vi "Main VERSION 2.0.vi"() -> ()   [LabVIEW 2017]
doc: "This Continuous Measurement sample project is based on the Queued Message Handler template.\n\nThe Event Handling Loop generates messages based on user interface actions.\n\nThe Message Handling Loop processes messages generated by the Event Handling Loop, or by other messages. There are also Acquisition and Logging message handling loop subVIs, and a chart updating loop."
uses:
  support/libs/Signal Selector/Selection Folder/Selection.xctl
  <vilib>/Math Plots/3D Math Plots/3D Surface/3D Surface XCtrl/3D Surface.xctl
  <vilib>/Math Plots/3D Math Plots/3D Surface/3D Surface Datatype/3D Surface Datatype.lvclass
  controls/UI Data.ctl
  support/libs/PMU Buffer/Buffer DATA cluster.ctl
  controls/UI State.ctl
  acquisition/Acquisition Settings.ctl
  acquisition/Acquisition State.ctl
  support/libs/CSV Reader/Mode CSV reader.ctl
  logging/Logging Configuration.ctl
  logging/Logging State.ctl
  support/libs/PMU Buffer/Buffer Settings.ctl
  processing/Processing Settings.ctl
  processing/Display Data B.ctl
  processing/Display Data A.ctl
  <vilib>/Math Plots/3D Math Plots/3D Plot/3D Plot Datatype/3D Plot Datatype.lvclass
  <vilib>/Utility/error.llb/DialogType.ctl
  support/libs/PMU Buffer/Buffer state.ctl
  support/settings/Settings.ctl
  b850246f-c621-4cc8-8cdb-6c63488b8d16.vi
  d6c7b380-5ef8-42a0-a533-ce26cb609579.vi
  5953c9e4-e6ed-48ce-a3e3-f4074e595e54.vi
  308fbb3a-e3c1-4651-8528-14e79cd65b6c.vi
  fb94752c-021c-42e0-8cca-361a15baff7d.vi
  17f702fa-b3ef-4227-89b6-1808d4fdff79.vi
  support/Message Queue/Enqueue Message (Single).vi
  <vilib>/S3DK/PMU Recorder Light/PRL Channel Selector.vi
  support/settings/Get Config File Path.vi
  <vilib>/Utility/xml.llb/Read From XML File.vi
  <vilib>/Utility/xml.llb/Read From XML File(string).vi
  <vilib>/Utility/xml.llb/Write to XML File.vi
  <vilib>/Utility/xml.llb/Write to XML File(string).vi
  <vilib>/Utility/error.llb/Error Cluster From Error Code.vi
  <vilib>/ErrorRing/Error Ring.xnode
  acquisition/Acquisition.lvlib
  logging/Logging.lvlib
  support/User Event - Stop/User Event - Stop.lvlib
  support/Message Queue/Message Queue.lvlib
  support/settings/Settings Dialog.vi
  support/settings/Settings.lvlib
  processing/Processing.lvlib
  support/libs/PMU Buffer/PMU data buffer.lvlib
  <vilib>/S3DK/PMU Recorder Light/PMU Recorder Light.lvlib
  support/libs/Signal Selector/Signal Selector.lvlib
panel:
  in  "Data Selector":bool
  in  "PRL Visible":bool
  out "Display 2":bool
  out "Buffer Active":bool
  out "Config File":bool
  out "Connected":bool
  out "Error":bool
  out "Processing":bool=TRUE
  out "Display":bool
  out "Acquisition":bool=TRUE
  out "Events":bool=TRUE
  out "Buffer":bool
  out "UI Control":bool
  in  "Tab Control":T1(tab)
  out "ARMA Transfer Function":picture
  out "Critical Damping [%]":dbl
  out "Critical Frequency [Hz]":dbl
  out "Estimated Complex Plane":cluster{dbl[], dbl[]}(graph)
  out "Damping ratio evolution":dbl[][](graph)
  out "Real-time data":waveform(dbl)(graph)={"t0"=timestamp(3467964116.0127993 s since 1904-01-01), "dt"=0.02, "Y"=array[30000 elements]}
  out "Preprocessed data":waveform(dbl)(graph)={"t0"=timestamp(3467964116.0127993 s since 1904-01-01), "dt"=0.2, "Y"=array[3000 elements]}
  out "Spectrogram":refnum<class "3D Plot Datatype.lvclass">[](xcontrol)
  out "Spectrum":cluster{"f0":dbl, "df":dbl, "S(f)":dbl[]}(graph)={"f0"=0.0, "df"=0.0048828125, "S(f)"=[]}
  out "Picture 9":picture
  out "Picture 8":picture
  out "Picture 7":picture
  out "Picture 6":picture
  out "Picture 5":picture
  out "Picture 4":picture
  out "Picture 3":picture
  out "Picture 2":picture
  out "Picture 1":picture
  out "Std of Damping":dbl[](array[numeric])
  out "Mean Damping [%]":dbl[](array[numeric])
  out "Frequency[Hz]":dbl[](array[numeric]) format="%.4f"
  out "Damping Ratio [%]":dbl[](array[numeric]) format="%.4f"
  out "Complex Poles":cdb[](array[numeric]) format="%.4f"
  in  "Selection":cluster{"Type":T2, "Index(es)":i32[]}[](xcontrol)
  in  "Settings":bool
  in  "Start":bool
  in  "Stop":bool
  out "Status":string
  in  "Exit":bool
  # "Continuous Measurement Data Logger"
  # "MA\n_______\n\n   AR"
  # "If you hit the bottom button, you will see the same chart as the one \non the Spectrum graph"
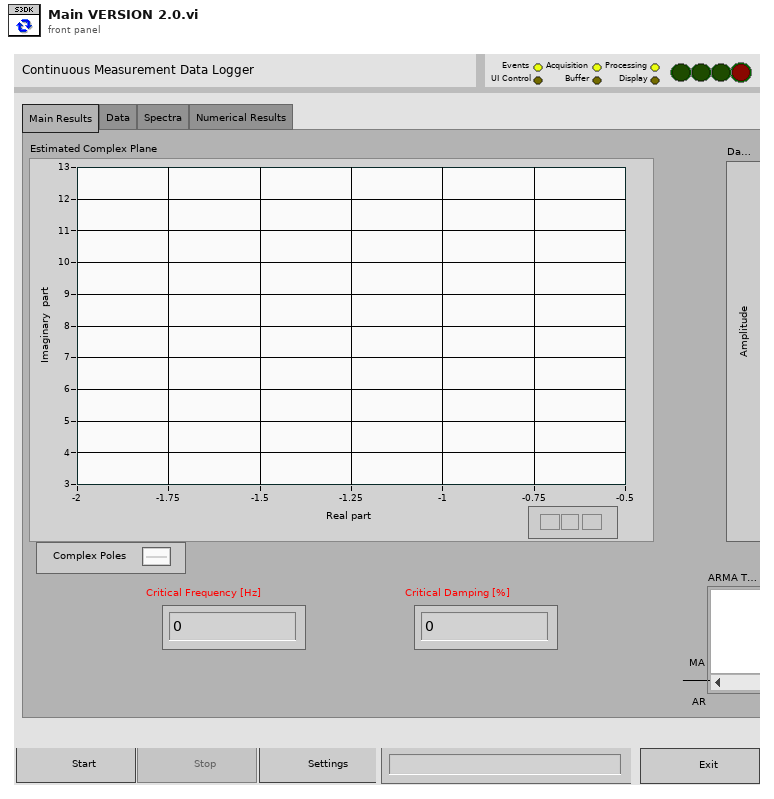
[diagram p1: front panel]
types:
  T1 = enum32{"Main Results", "Data", "Spectra", "Numerical Results"}
  T2 = typedef "Selection.xctl/Signal types.ctl" = enum16{"Disable", "Frequency", "Phasor Mag", "Phasor Ang", "Angle Diff", "P", "Q"}
  T3 = typedef "Display Data A.ctl" = cluster{"Real-time data":waveform(dbl), "Preprocessed data":waveform(dbl), "ARMA Transfer Function":picture, "Spectrogram":refnum<class "3D Plot Datatype.lvclass">[], "Spectrum":cluster{"f0":dbl, "df":dbl, "S(f)":dbl[]}, "Parcel Length (SDK or Simulation)":i32}
  T4 = typedef "Display Data B.ctl" = cluster{"Damping ratio evolution":dbl[][], "Estimated Complex Plane":cluster{dbl[], dbl[]}, "Critical Frequency [Hz]":dbl, "Critical Damping [%]":dbl, " Complex Poles":cdb[], "Damping Ratio [%]":dbl[], " Frequency[Hz]":dbl[], "Mean Damping [%]":dbl[], "Pictures":picture[], "Std of Damping":dbl[]}
  T5 = typedef "Processing.lvlib/Processing Settings.ctl" = cluster{"Settings":string, "Parameters":T6, "Refresh Rate":u32}
  T6 = typedef "PMU data buffer.lvlib/Buffer Settings.ctl" = cluster{"Index":i32, "Size":i32, "Samples":i32, "Ordered ?":bool}
  T7 = typedef "Logging.lvlib/Logging Configuration.ctl" = cluster{"Logging State":T8, "Settings":string, "Buffer":T6}
  T8 = typedef "Logging.lvlib/Logging State.ctl" = enum16{"Idle", "Logging"}
  T9 = typedef "Acquisition.lvlib/Acquisition Settings.ctl" = cluster{"State":T10, "Settings":string, "Online":bool, "S3DK":cluster{"Signals":cluster{"Phasor":string[], "Analog":string[], "Digital":string[]}}, "CSV":cluster{"Index":i32, "Parcel Length":i32, "EOF?":bool, "Config":cluster{"Mode":T11, "delimiter (\\t)":string, "Path":path, "Rectangular?":bool}}}
  T10 = typedef "Acquisition.lvlib/Acquisition State.ctl" = enum16{"Idle", "Idle S3DK", "Acquiring S3DK", "Idle CSV", "Acquiring CSV"}
  T11 = typedef "Mode CSV reader.ctl" = enum16{"Full timestamp", "Relative Time", "Seconds Time", "Nanoseconds Time"}
  T12 = typedef "UI State.ctl" = enum16{"Idle", "Acquiring and Logging", "Waiting for Exit", "Waiting for Exit (Acq Stopped)", "Waiting for Exit (Log Stopped)", "Waiting for Stop", "Waiting for Stop (Acq Stopped)", "Waiting for Stop (Log Stopped)"}
  T13 = typedef "PMU data buffer.lvlib/Buffer DATA cluster.ctl" = cluster{timestamp, csg[], sgl[]}
  T14 = typedef "UI Data.ctl" = cluster{"Start Ref":refnum<vi>, "Stop Ref":refnum<vi>, "Settings Ref":refnum<vi>, "Exit Ref":refnum<vi>, "Status Ref":refnum<vi>, "Data Ref":refnum<vi>, "Data Selector":refnum<vi>, "PRL Visible":refnum<vi>}
  T15 = typedef "Message Queue.lvlib/All Message Queues.ctl" = cluster{"UI":refnum<queue>, "Acquisition":refnum<queue>, "Logging":refnum<queue>, "Processing":refnum<queue>}
  T16 = typedef "PMU data buffer.lvlib/Buffer state.ctl" = enum16{"Init", "Change Size", "Flush", "Exit", "Add", "Get", "Hist_Toggle", "Add_Serv"}
  T17 = typedef "DialogType.ctl" = u16
  T18 = typedef "Mode Est Processing Settings.ctl" = cluster{"Low-Pass Filter Order":i32, "Downsampling Ratio":dbl, "LPF Cut-off Frequency [Hz]":dbl, "Sampling Frequency (Hz)":dbl, "Parcel Length":i32, "Detrend Cut-off Frequency (Hz)":dbl, "AR Order":i32, "MA Order ":i32, "Lower Frequency [Hz]":dbl, "Upper Frequency [Hz]":dbl, "Upper Damping [%]":dbl, "Lower Damping [%]":dbl, "Std Threshold":dbl, "Length of Spectra [s]":dbl, "Refresh Rate [s]":i32, "Number of critical modes":i32}
  T19 = typedef "PMU data buffer.lvlib/Buffer DATA OUT ordered.ctl" = cluster{"Timestamp":timestamp[], "Phasor":csg[][], "Analog":sgl[][]}
  T20 = enum16{"Run", "Startup", "Get Status", "Pause", "Continue", "Shutdown", "Abort", "Open Panel", "Close Panel"}
  T21 = enum32{"Invalid", "Standard", "Closed", "Hidden", "Minimized", "Maximized"}
  T22 = typedef "Settings.lvlib/Settings.ctl" = cluster{"Acquisition":T9, "Logging":T7, "Processing":T5}
  T23 = cluster{"[0]":variant, "[1]":variant, "[2]":variant}
  T24 = typedef "Terminal Data.ctl" = cluster{"Spreadsheet":path, "Terminal ID":u32, "Terminal Name":string}
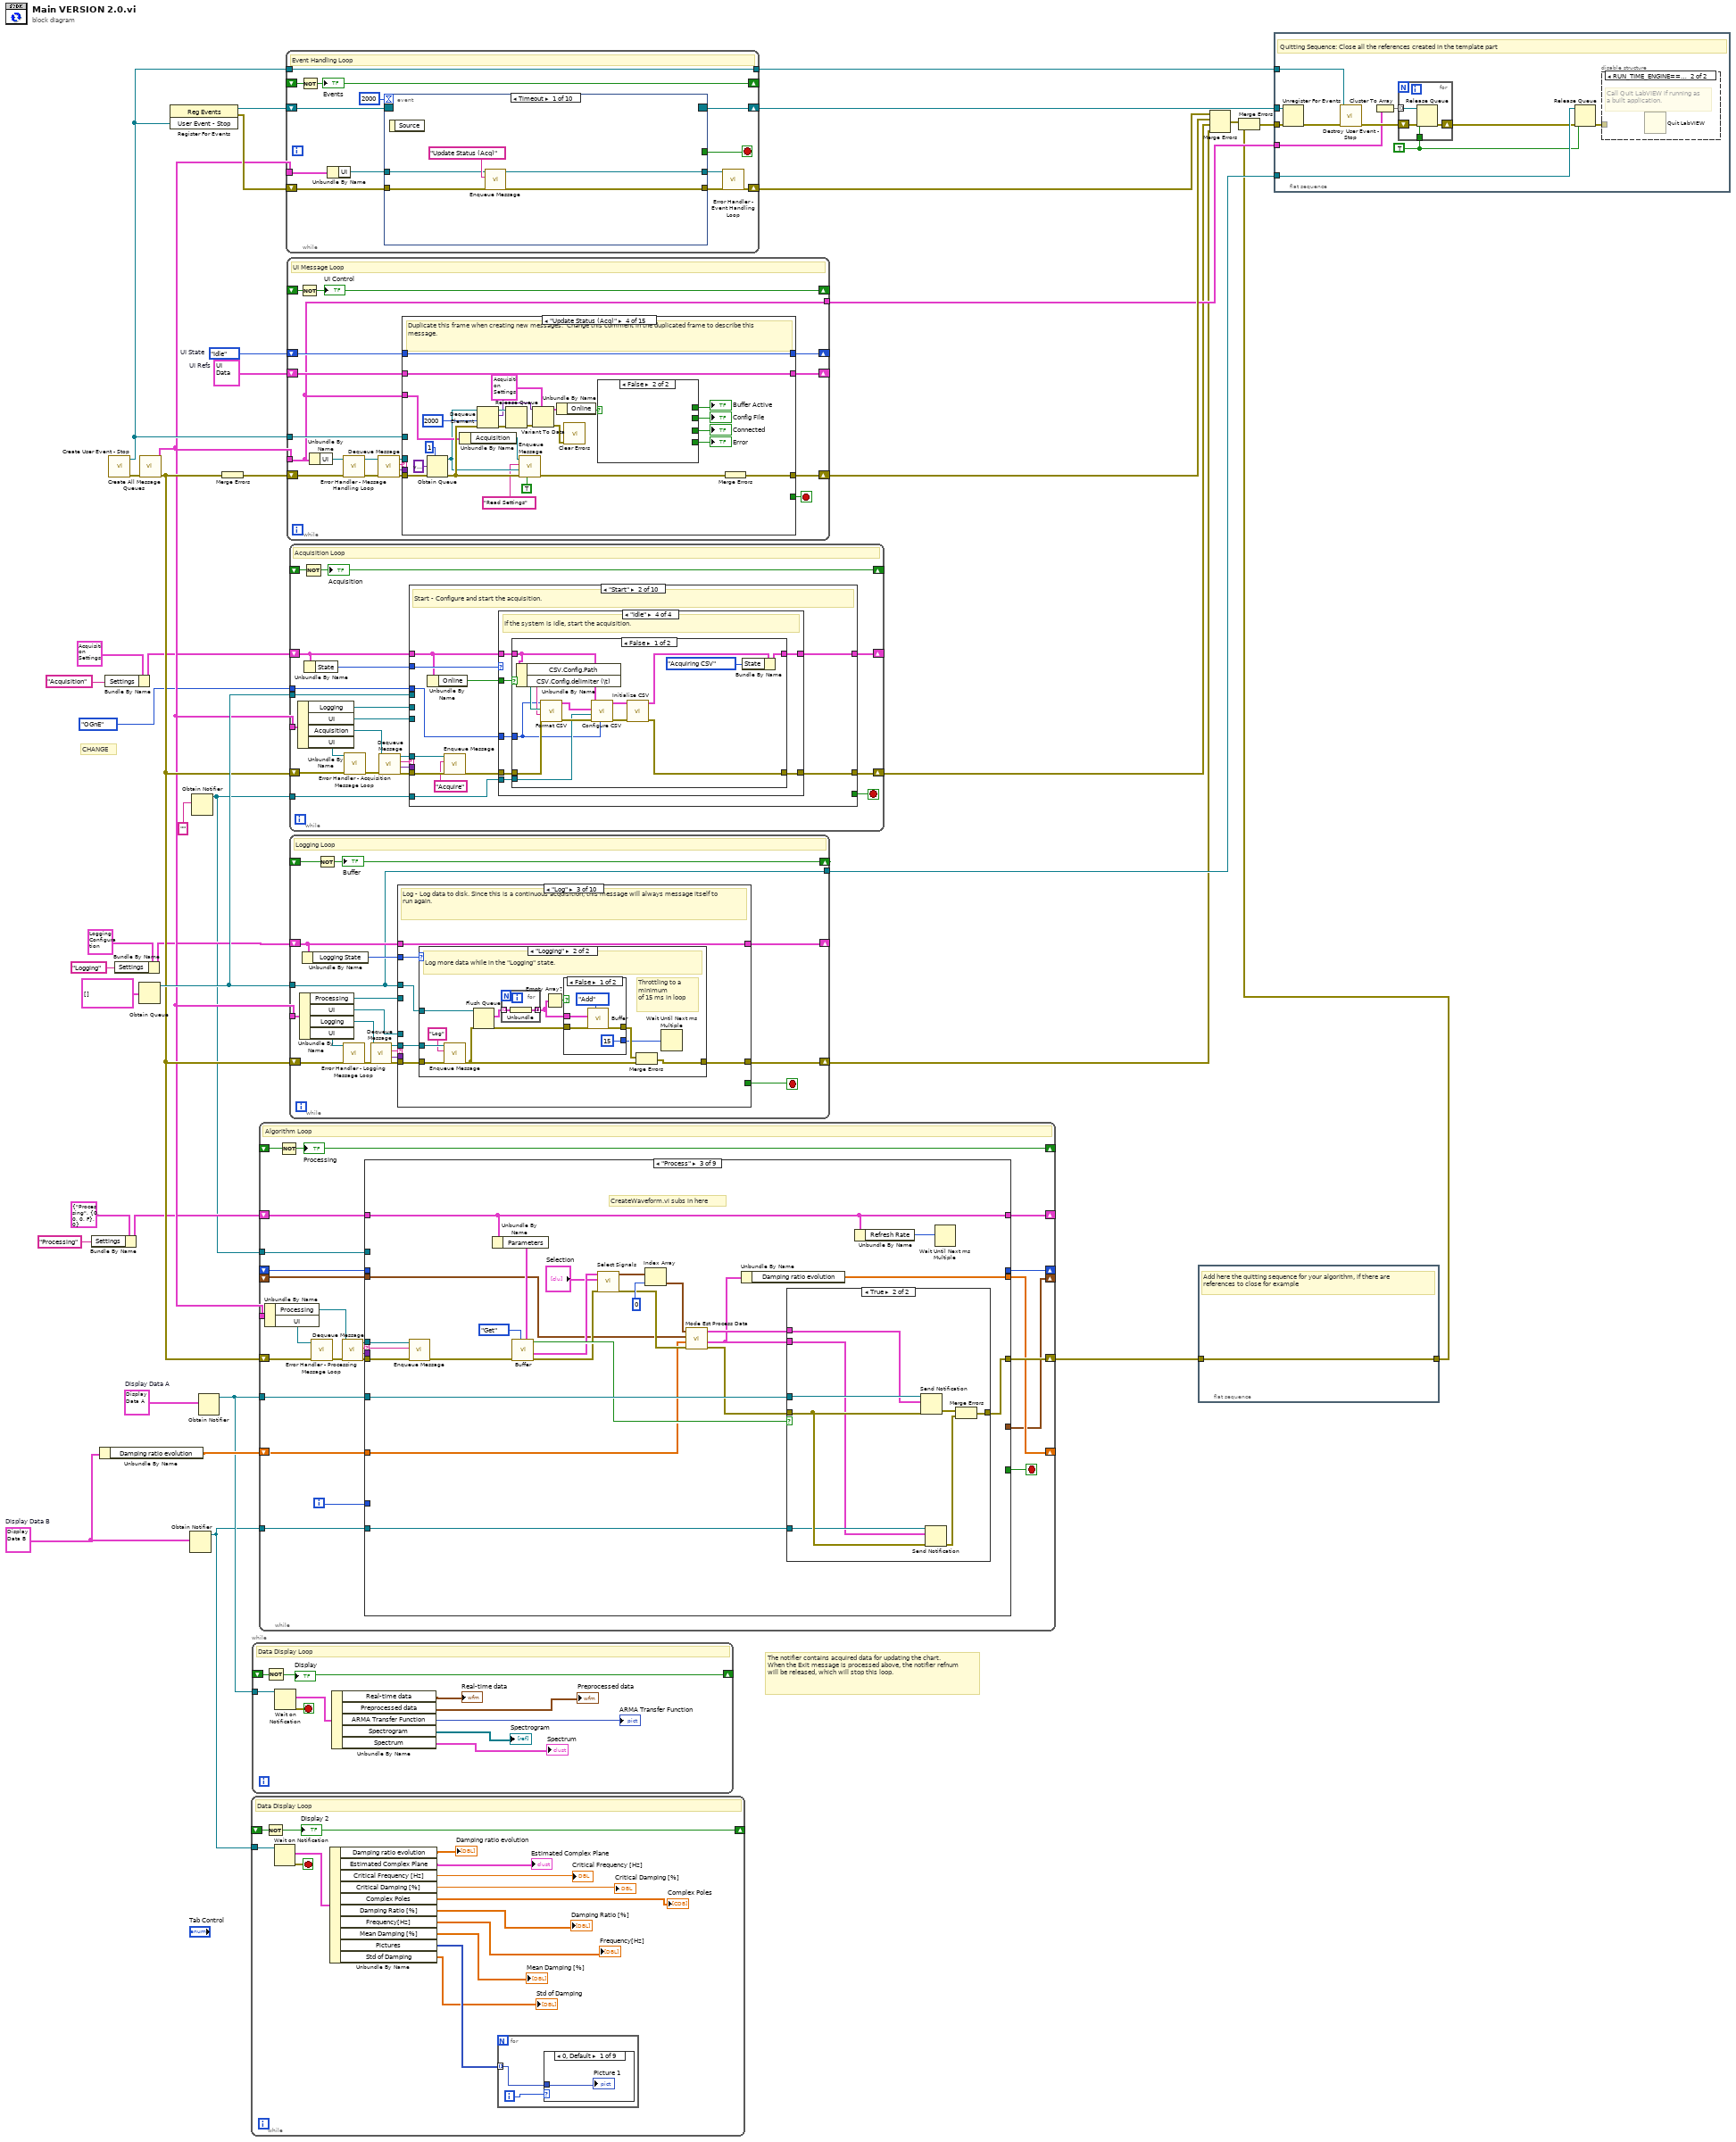
[diagram p0: block diagram]
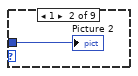
[diagram p2: hidden frame]
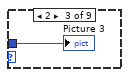
[diagram p3: hidden frame]
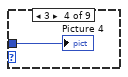
[diagram p4: hidden frame]
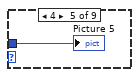
[diagram p5: hidden frame]
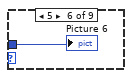
[diagram p6: hidden frame]
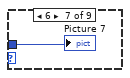
[diagram p7: hidden frame]
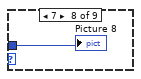
[diagram p8: hidden frame]
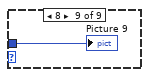
[diagram p9: hidden frame]
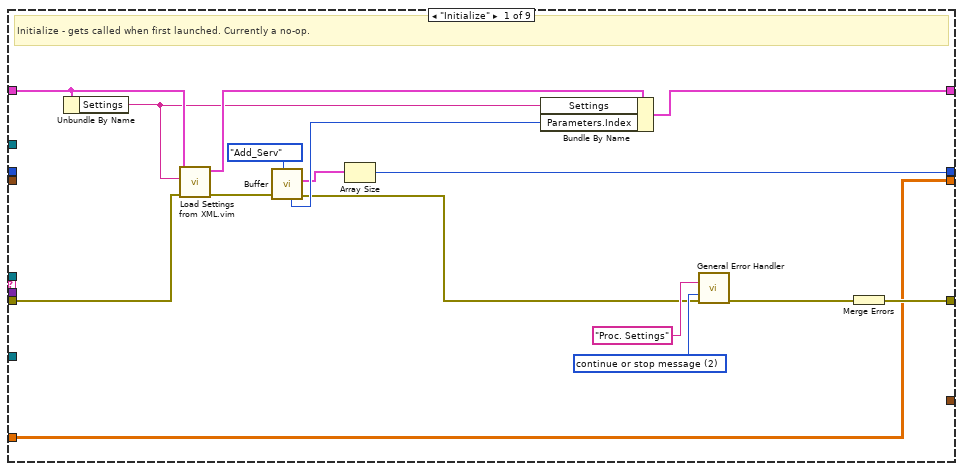
[diagram p11: hidden frame]
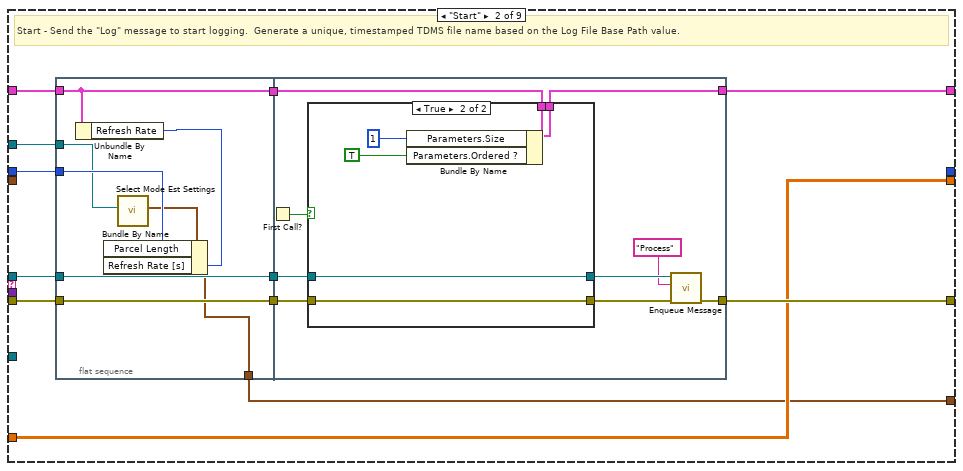
[diagram p12: hidden frame]
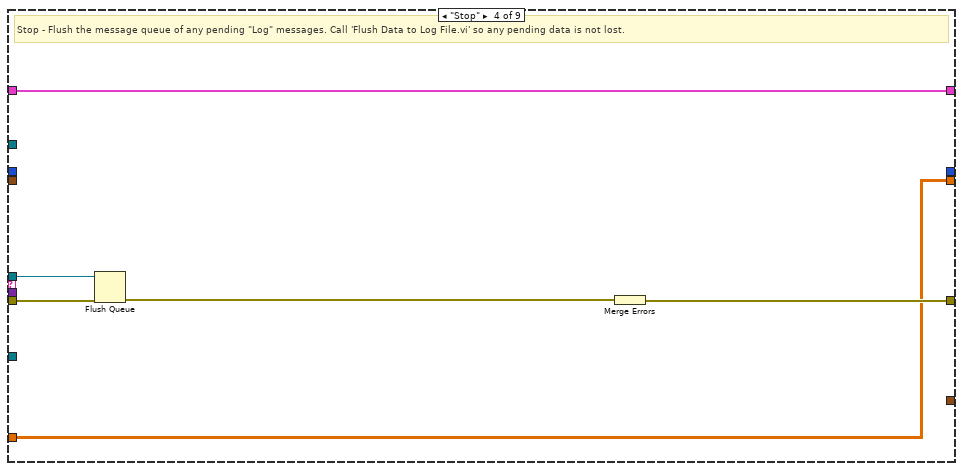
[diagram p15: hidden frame]
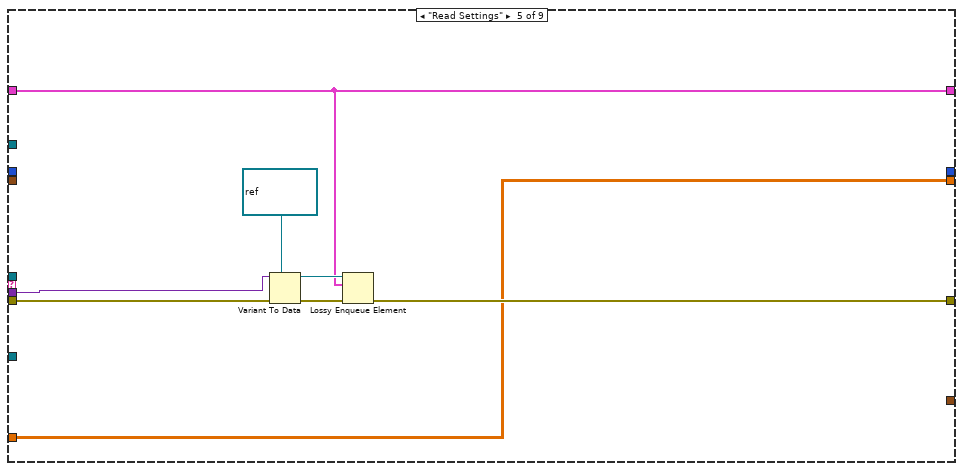
[diagram p16: hidden frame]
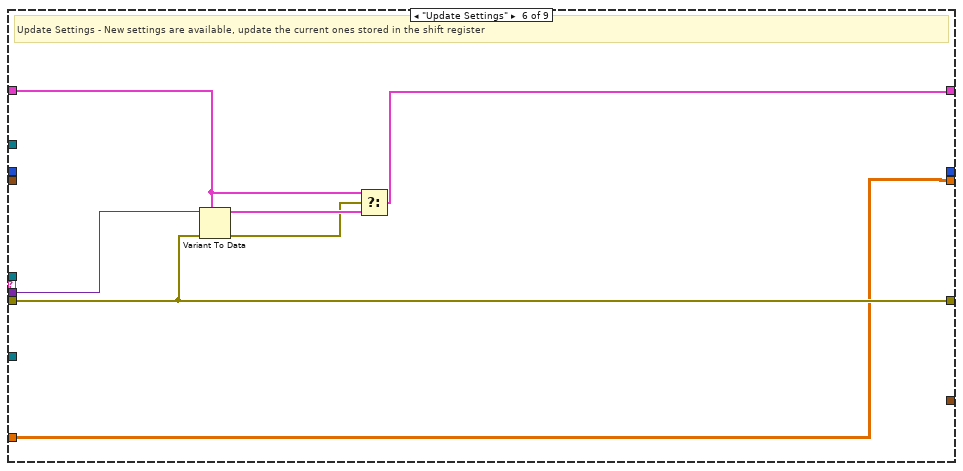
[diagram p17: hidden frame]
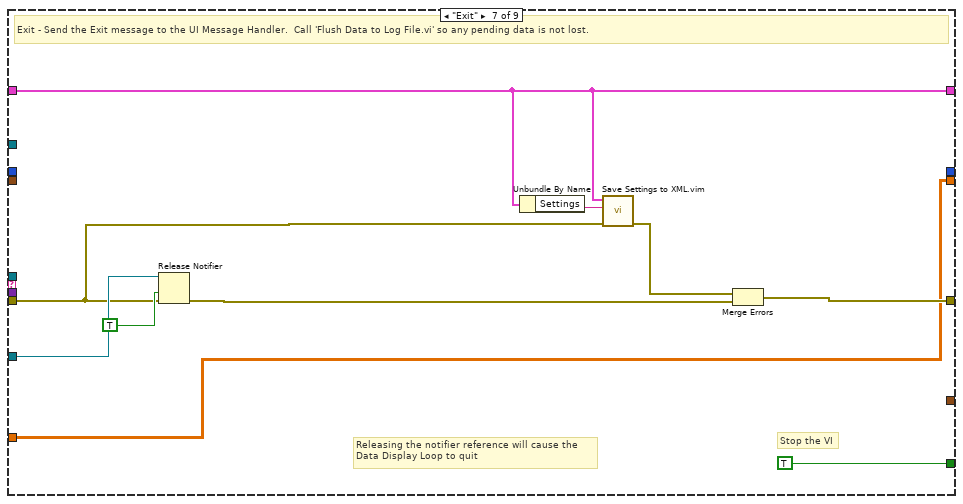
[diagram p18: hidden frame]
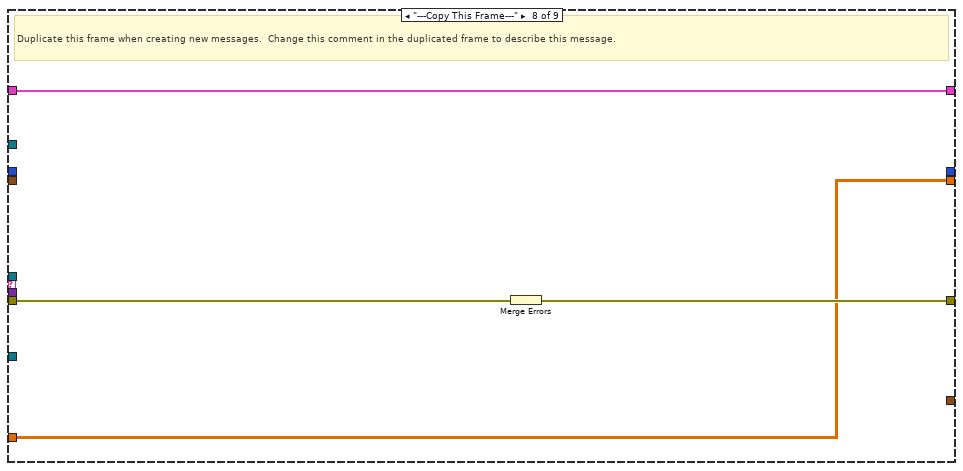
[diagram p19: hidden frame]
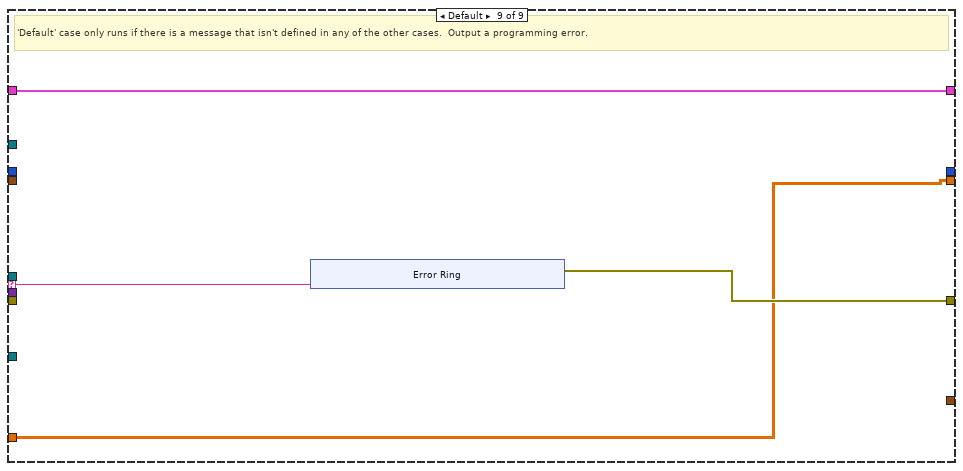
[diagram p20: hidden frame]
diagram:
  w8 = T3 {"Real-time data"={"t0"=timestamp(3467964116.0127993 s since 1904-01-01), "dt"=0.02, "Y"=array[30000 elements]}, "Preprocessed data"={"t0"=timestamp(3467964116.0127993 s since 1904-01-01), "dt"=0.2, "Y"=array[3000 elements]}, "ARMA Transfer Function"=bytes[0], "Spectrogram"=[refnum], "Spectrum"={"f0"=0.0, "df"=0.0048828125, "S(f)"=[]}, "Parcel Length (SDK or Simulation)"=30000}  # Display Data A
  w6 = T4 {"Damping ratio evolution"=[], "Estimated Complex Plane"={[], []}, "Critical Frequency [Hz]"=0.0, "Critical Damping [%]"=0.0, " Complex Poles"=[0.0+0.0i, 0.0+0.0i, 0.0+0.0i], "Damping Ratio [%]"=[0.0, 0.0, 0.0], " Frequency[Hz]"=[0.0, 0.0, 0.0], "Mean Damping [%]"=[0.0, 0.0, 0.0], "Pictures"=[bytes[260130], bytes[260130], bytes[260130]], "Std of Damping"=[0.0, 0.0, 0.0]}  # Display Data B
  w38 = UI_State."Idle"  # UI State
  w39 = T14 {"Start Ref"=refnum, "Stop Ref"=refnum, "Settings Ref"=refnum, "Exit Ref"=refnum, "Status Ref"=refnum, "Data Ref"=refnum, "Data Selector"=refnum, "PRL Visible"=refnum}  # UI Refs
  # "CHANGE"
  # "The notifier contains acquired data for updating the chart. When the Exit message is processed above, the notifier refnum will be released, which will stop this loop."
  n1 = Bundle By Name(cluster=T5 {"Settings"="Processing", "Parameters"={"Index"=0, "Size"=0, "Samples"=0, "Ordered ?"=FALSE}, "Refresh Rate"=0} ("Processing Settings"), "Settings"="Processing") -> (w10:T5)
  n2 = Unbundle By Name(w6) -> ("Damping ratio evolution"=w5:dbl[][])
  n3 = Bundle By Name(cluster=T9 {"State"=enum."Idle S3DK", "Settings"="Acquisition", "Online"=FALSE, "S3DK"={"Signals"={"Phasor"=[], "Analog"=[], "Digital"=[]}}, "CSV"={"Index"=0, "Parcel Length"=0, "EOF?"=FALSE, "Config"={"Mode"=enum."Full timestamp", "delimiter (\\t)"=",", "Path"=path "", "Rectangular?"=TRUE}}} ("Data Cluster"), "Settings"="Acquisition") -> (w14:T9)
  n4 = call "Create User Event - Stop.vi"() -> ("error out"=w40:errorcluster, "User Event - Stop"=w22:refnum<user-event>)  [unwired: 10 in]
  n5 = Bundle By Name(cluster=T7 {"Logging State"=enum."Idle", "Settings"="Logging", "Buffer"={"Index"=0, "Size"=15000, "Samples"=0, "Ordered ?"=FALSE}} ("Logging Configuration"), "Settings"="Logging") -> (w12:T7)
  n6 = Obtain Queue(element data type=T13[] []) -> (queue out=w34:refnum<queue>)  [unwired: 4 in, 2 out]
  n7 = call "Create All Message Queues.vi"("error in (no error)"=w40) -> ("error out"=w16:errorcluster, "Message Queues out"=w15:T15)  [unwired: 9 in]
  n8 = register-events(w22) -> (reference out=w36:refnum<event-registration>, error out=w17:errorcluster)  [unwired: 2 in]
  n9 = Obtain Notifier(notification data type=w6) -> (notifier out=w1:refnum<notifier>)  [unwired: 3 in, 2 out]
  n10 = Obtain Notifier(notification data type="" ("String")) -> (notifier out=w3:refnum<notifier>)  [unwired: 3 in, 2 out]
  n11 = Obtain Notifier(notification data type=w8) -> (notifier out=w2:refnum<notifier>)  [unwired: 3 in, 2 out]
  n12 = Merge Errors(w16) -> (w35:errorcluster)
  n13 = while "Data Display Loop" {
    tunnel: w1 -> [w55]
    shift-right: [w50] -> _
    shift-left: _ -> [w53]
    stop <- w54 stop-if-true
    # "Data Display Loop"
    n14 = Not(x=w53) -> (.not. x?=w50:bool)
    "Display 2" <- w50
    n15 = Wait on Notification(notifier=w55) -> (notification=w52:T4, error out=w54:errorcluster)  [unwired: 3 in, 2 out]
    n16 = Unbundle By Name(w52) -> ("Damping ratio evolution"=→"Damping ratio evolution":dbl[][], "Estimated Complex Plane"=→"Estimated Complex Plane":cluster{dbl[], dbl[]}, "Critical Frequency [Hz]"=→"Critical Frequency [Hz]":dbl, "Critical Damping [%]"=→"Critical Damping [%]":dbl, "Complex Poles"=→"Complex Poles":cdb[], "Damping Ratio [%]"=→"Damping Ratio [%]":dbl[], "Frequency[Hz]"=→"Frequency[Hz]":dbl[], "Mean Damping [%]"=→"Mean Damping [%]":dbl[], "Pictures"=w51:picture[], "Std of Damping"=→"Std of Damping":dbl[])
    n17 = for {
      tunnel: w51 -> [w56] mode=indexing
      i -> [w57]
      n18 = case shown="0, Default" w57 {
        tunnel: w56 -> [w58 w59 w60 w61 w62 w63 w64 w65 w66]
        frame 0, Default {
          "Picture 1" <- w58
        }
        frame 1 {
          "Picture 2" <- w59
        }
        frame 2 {
          "Picture 3" <- w60
        }
        frame 3 {
          "Picture 4" <- w61
        }
        frame 4 {
          "Picture 5" <- w62
        }
        frame 5 {
          "Picture 6" <- w63
        }
        frame 6 {
          "Picture 7" <- w64
        }
        frame 7 {
          "Picture 8" <- w65
        }
        frame 8 {
          "Picture 9" <- w66
        }
      }
    }
  }
  n19 = while "Data Display Loop" {
    tunnel: w2 -> [w76]
    shift-right: [w72] -> _
    shift-left: _ -> [w74]
    stop <- w75 stop-if-true
    # "Data Display Loop"
    n20 = Not(x=w74) -> (.not. x?=w72:bool)
    "Display" <- w72
    n21 = Wait on Notification(notifier=w76) -> (notification=w73:T3, error out=w75:errorcluster)  [unwired: 3 in, 2 out]
    n22 = Unbundle By Name(w73) -> ("Real-time data"=→"Real-time data":waveform(dbl), "Preprocessed data"=→"Preprocessed data":waveform(dbl), "ARMA Transfer Function"=→"ARMA Transfer Function":picture, "Spectrogram"=→"Spectrogram":refnum<class "3D Plot Datatype.lvclass">[], "Spectrum"=→"Spectrum":cluster{"f0":dbl, "df":dbl, "S(f)":dbl[]})
  }
  n23 = while {
    tunnel: w2 -> [w91]
    shift-right: [w101] -> _
    shift-left: _ -> [w100]
    shift-right: [w93] -> _
    shift-left: w10 -> [w94]
    tunnel: w15 -> [w99]
    shift-right: [w88] -> w20
    shift-left: w16 -> [w87]
    tunnel: w1 -> [w84]
    shift-right: [w83] -> _
    shift-left: w5 -> [w82]
    shift-right: [w81] -> _
    shift-left: _ -> [w80]
    shift-right: [w79] -> _
    shift-left: _ -> [w78]
    tunnel: w3 -> [w77]
    i -> [w90]
    stop <- w92 stop-if-true
    # "Algorithm Loop"
    n24 = Unbundle By Name(w99) -> ("Processing"=w89:refnum<queue>, "UI"=w85:refnum<queue>)
    n25 = Not(x=w100) -> (.not. x?=w101:bool)
    "Processing" <- w101
    n26 = call "Error Handler - Processing Message Loop.vi"("error in (no error)"=w87, "Message Queue"=w85) -> ("dup error in"=w86:errorcluster)  [unwired: 8 in, 1 out]
    n27 = call "Dequeue Message.vi"("error in (no error)"=w86, "Message Queue"=w89) -> ("error out"=w96:errorcluster, "Message Data"=w95:variant, "Message"=w97:string, "dup Message Queue"=w98:refnum<queue>)  [unwired: 6 in]
    n28 = case "Message Cases" shown="\"Process\"" w97 {
      selector: w97 -> [_ _ w180 _ _ _ _ _ w227]
      tunnel: w98 -> [_ w128 w179 w192 _ _ _ _ _]
      tunnel: w96 -> [w110 w129 w166 w193 w198 w205 w212 w224 _]
      tunnel: w94 -> [w115 w127 w174 w195 w199 w207 w216 w223 w228]
      tunnel: [w111 w126 w174 w195 w199 w206 w216 w223 w228] -> w93
      tunnel: [_ _ _ _ _ _ TRUE _ _] -> w92
      tunnel: w95 -> [_ _ _ _ w200 w210 _ _ _]
      tunnel: [w108 w125 w169 w194 w197 w205 w219 w222 w226] -> w88
      tunnel: w91 -> [_ _ w177 _ _ _ w218 _ _]
      tunnel: w90 -> [_ _ _ _ _ _ _ _ _]
      tunnel: w84 -> [_ _ w164 _ _ _ _ _ _]
      tunnel: [w104 w124 w158 w190 w196 w204 w211 w221 w225] -> w83
      tunnel: w82 -> [w104 w124 w157 w190 w196 w204 w211 w221 w225]
      tunnel: [_ w119 _ _ _ _ _ _ _] -> w81
      tunnel: w80 -> [_ _ w156 _ _ _ _ _ _]
      tunnel: [w102 _ _ _ _ _ _ _ _] -> w79
      tunnel: w78 -> [_ w120 _ _ _ _ _ _ _]
      tunnel: w77 -> [_ w118 _ _ _ _ _ _ _]
      frame "Initialize" {
        w117 = T17 2 items=["no dialog", "OK message", "continue or stop message", "OK message + warnings", "continue/stop + warnings"] ("type of dialog (OK msg:1)")
        # "Initialize - gets called when first launched. Currently a no-op."
        n29 = Unbundle By Name(w115) -> ("Settings"=w107:string)
        n30 = call "Load Settings from XML.vim"("error in (no error)"=w110, "Settings File Name"=w107, "Settings In"=w115) -> ("error out"=w112:errorcluster, "Settings Out"=w113:T5)  [unwired: 7 in]
        n31 = call "Buffer.vi"("Mode"=Buffer_state."Add_Serv", "Error IN"=w112) -> ("Error OUT"=w105:errorcluster, "DATA OUT"=w103:T13[], "Index"=w114:i32)  [unwired: 5 in, 2 out]
        n32 = Array Size(array=w103) -> (size(s)=w102:i32)
        n33 = Bundle By Name(cluster=w113, "Settings"=w107, "Parameters.Index"=w114) -> (w111:T5)
        n34 = call <vilib>:"General Error Handler.vi"("[error source] (\" \")"="Proc. Settings" ("[error source] (\" \")"), "type of dialog (OK msg:1)"=w117, "error in (no error)"=w105) -> ("error out"=w106:errorcluster)  [unwired: 8 in, 4 out]
        n35 = Merge Errors(w106) -> (w108:errorcluster)
      }
      frame "Start" {
        # "Start - Send the \"Log\" message to start logging.  Generate a unique, timestamped TDMS file name based on the Log File Base Path value."
        n36 = flat-sequence {
          tunnel: w127 -> [w132]
          tunnel: w128 -> [w136]
          tunnel: w129 -> [w137]
          tunnel: [w137] -> w123
          tunnel: [w136] -> w122
          tunnel: [w132] -> w121
          tunnel: w120 -> [w135]
          tunnel: [w133] -> w119
          tunnel: w118 -> [w130]
          tunnel: [w143] -> w126
          tunnel: [w141] -> w125
          tunnel: w123 -> [w146]
          tunnel: w122 -> [w145]
          tunnel: w121 -> [w144]
          frame #0 {
            n37 = Unbundle By Name(w132) -> ("Refresh Rate"=w131:u32)
            n38 = call "Select Mode Est Settings.vi"("notifier"=w130) -> ("Mode Estimator Processing Settings out"=w134:T18)  [unwired: 10 in]
            n39 = Bundle By Name(cluster=w134, "Parcel Length"=w135, "Refresh Rate [s]"=w131) -> (w133:T18)
          }
          frame #1 {
            n40 = First Call?() -> (First Call?: T/F=w138:bool)
            n41 = case shown="True" w138 {
              tunnel: w146 -> [w147 w150]
              tunnel: w145 -> [w148 w151]
              tunnel: w144 -> [w149 w155]
              tunnel: [w149 w154] -> w143
              tunnel: [w147 w150] -> w142
              tunnel: [w148 w151] -> w140
              frame False {
              }
              frame True {
                n42 = Bundle By Name(cluster=w155, "Parameters.Size"=1 ("Params Energy.Size"), "Parameters.Ordered ?"=TRUE ("Params Energy.Ordered ?")) -> (w154:T5)
              }
            }
            n43 = call-poly "Enqueue Message.vi"("error in (no error)"=w142, "Message"="Process", "Message Queue"=w140) -> ("error out"=w141:errorcluster)  [unwired: 7 in, 1 out]
          }
        }
      }
      frame "Process" {
        # "CreateWaveform.vi subs in here"
        n44 = call-poly "Enqueue Message.vi"("error in (no error)"=w166, "Message"=w180, "Message Queue"=w179) -> ("error out"=w173:errorcluster)  [unwired: 7 in, 1 out]
        n45 = Unbundle By Name(w174) -> ("Parameters"=w168:T6)
        n46 = call "Buffer.vi"("Parameters"=w168, "Mode"=Buffer_state."Get", "Error IN"=w173) -> ("Error OUT"=w171:errorcluster, "Output"=w172:T19, "New Element ?"=w176:bool)  [unwired: 4 in, 2 out]
        n47 = call "Select Signals.vi"("Error In"=w171, "Selection"="Selection", "DATA IN"=w172) -> ("Error Out"=w163:errorcluster, "Array"=w170:waveform(dbl)[])  [unwired: 6 in, 1 out]
        n48 = Index Array(array=w170, index=0) -> (element=w161:waveform(dbl))
        n49 = call "Mode Est Process Data.vi"("error in (no error)"=w163, "Damping Ratio History"=w157, "Mode Estimator Processing Settings"=w156, "Waveform in"=w161) -> ("error out"=w162:errorcluster, "Display Data B"=w159:T4, "Display Data A"=w160:T3)  [unwired: 5 in]
        n50 = Unbundle By Name(w159) -> ("Damping ratio evolution"=w158:dbl[][])
        n51 = case shown="True" w176 {
          tunnel: w177 -> [_ w189]
          tunnel: w162 -> [w181 w188]
          tunnel: [w181 w186] -> w169
          tunnel: w164 -> [_ w187]
          tunnel: w160 -> [_ w183]
          tunnel: w159 -> [_ w182]
          frame False {
          }
          frame True {
            n52 = Send Notification(notification=w183, notifier=w189, error in (no error)=w188) -> (error out=w184:errorcluster)  [unwired: 1 out]
            n53 = Send Notification(notification=w182, notifier=w187, error in (no error)=w188) -> (error out=w185:errorcluster)  [unwired: 1 out]
            n54 = Merge Errors(w184, w185) -> (w186:errorcluster)
          }
        }
        n55 = Unbundle By Name(w174) -> ("Refresh Rate"=w175:u32)
        n56 = Wait Until Next ms Multiple(millisecond multiple=w175) -> ()  [unwired: 1 out]
      }
      frame "Stop" {
        # "Stop - Flush the message queue of any pending \"Log\" messages. Call 'Flush Data to Log File.vi' so any pending data is not lost."
        n57 = Flush Queue(queue=w192, error in (no error)=w193) -> (error out=w191:errorcluster)  [unwired: 2 out]
        n58 = Merge Errors(w191) -> (w194:errorcluster)
      }
      frame "Read Settings" {
        n59 = Variant To Data(error in=w198, type=refnum<queue> refnum ("queue out"), Variant=w200) -> (data=w201:refnum<queue>, error out=w202:errorcluster)
        n60 = Lossy Enqueue Element(queue=w201, element=w199, error in (no error)=w202) -> (error out=w197:errorcluster)  [unwired: 3 out]
      }
      frame "Update Settings" {
        # "Update Settings - New settings are available, update the current ones stored in the shift register"
        n61 = Variant To Data(error in=w205, type=w207, Variant=w210) -> (data=w209:T5, error out=w208:errorcluster)
        n62 = Select(t=w207, s=w208, f=w209) -> (s? t:f=w206:T5)
      }
      frame "Exit" {
        # "Releasing the notifier reference will cause the \nData Display Loop to quit"
        # "Stop the VI"
        # "Exit - Send the Exit message to the UI Message Handler.  Call 'Flush Data to Log File.vi' so any pending data is not lost."
        n63 = Release Notifier(notifier=w218, force destroy? (F)=TRUE, error in (no error)=w212) -> (error out=w213:errorcluster)  [unwired: 2 out]
        n64 = Unbundle By Name(w216) -> ("Settings"=w217:string)
        n65 = call "Save Settings to XML.vim"("error in (no error)"=w212, "Settings File Name"=w217, "Settings In"=w216) -> ("error out"=w215:errorcluster)  [unwired: 8 in]
        n66 = Merge Errors(w215, w213) -> (w219:errorcluster)
      }
      frame "---Copy This Frame---" {
        # "Duplicate this frame when creating new messages.  Change this comment in the duplicated frame to describe this message."
        n67 = Merge Errors(w224) -> (w222:errorcluster)
      }
      frame Default {
        # "'Default' case only runs if there is a message that isn't defined in any of the other cases.  Output a programming error."
        n68 = xnode "Error Ring"("parameter 0"=w227) -> ("error out"=w226:errorcluster)
      }
    }
  }
  n69 = while {
    shift-right: [w247] -> w33
    shift-left: w36 -> [w248]
    tunnel: w15 -> [w237]
    shift-right: [w240] -> _
    shift-left: _ -> [w241]
    shift-right: [w245] -> w23
    shift-left: w17 -> [w238]
    tunnel: w22 -> [w236]
    tunnel: [w236] -> w21
    stop <- w246 stop-if-true
    # "Event Handling Loop"
    n70 = Not(x=w241) -> (.not. x?=w240:bool)
    "Events" <- w240
    n71 = Unbundle By Name(w237) -> ("UI"=w242:refnum<queue>)
    n72 = event shown="[0] Timeout" {
      selector: w248 -> [_ _ _ _ _ _ _ _ _ _]
      dyn-events: [_ _ _ _ _ _ _ _ _ _] -> w247
      timeout: 2000 -> [_ _ _ _ _ _ _ _ _ _]
      tunnel: [_ _ _ _ _ _ _ _ _ TRUE ("Discard?")] -> w246
      tunnel: w242 -> [w250 w257 w259 w263 w268 w271 w273 w280 w285 w297]
      tunnel: [w252 w255 _ w262 w266 _ w276 w278 w286 _] -> w244
      tunnel: [w249 w254 w258 w261 w267 w271 w272 w280 w285 w297] -> w243
      tunnel: w238 -> [w253 _ _ _ _ _ _ w279 w287 _]
      event Timeout {
        n73 = event-data() -> ()  [unwired: 1 in, 1 out]
        n74 = call-poly "Enqueue Message.vi"("error in (no error)"=w253, "Message"="Update Status (Acq)", "Message Queue"=w250) -> ("error out"=w252:errorcluster, "dup Message Queue"=w249:refnum<queue>)  [unwired: 7 in]
      }
      event "Start": Value Change {
        n75 = event-data() -> ()  [unwired: 1 in, 1 out]
        n76 = call-poly "Enqueue Message.vi"("Message"="Start", "Message Queue"=w257) -> ("error out"=w255:errorcluster, "dup Message Queue"=w254:refnum<queue>)  [unwired: 8 in]
      }
      event "Settings": Value Change {
        n77 = event-data() -> ()  [unwired: 1 in, 1 out]
        n78 = call-poly "Enqueue Message.vi"("Message"="Launch Settings Dialog", "Message Queue"=w259) -> ("dup Message Queue"=w258:refnum<queue>)  [unwired: 8 in, 1 out]
      }
      event "Stop": Value Change {
        n79 = event-data() -> ()  [unwired: 1 in, 1 out]
        n80 = call-poly "Enqueue Message.vi"("Message"="Stop", "Message Queue"=w263) -> ("error out"=w262:errorcluster, "dup Message Queue"=w261:refnum<queue>)  [unwired: 8 in]
      }
      event Panel Close? {
        # "Send the 'Confirm Quit' message if the user closes the panel of the VI. Discard the event so the 'Confirm Quit' message has a chance to run."
        n81 = event-data() -> ()  [unwired: 1 in, 1 out]
        n82 = call-poly "Enqueue Message.vi"("Priority Message? (F)"=TRUE, "Message"="Confirm Quit", "Message Queue"=w268) -> ("error out"=w266:errorcluster, "dup Message Queue"=w267:refnum<queue>)  [unwired: 7 in]
        n83 = event-data("Discard?"=TRUE) -> ()  [unwired: 1 in, 1 out]
      }
      event Application Instance Close {
        n84 = event-data() -> ()  [unwired: 1 in, 1 out]
      }
      event "Exit": Value Change {
        w274 = TRUE  # Priority Message
        # "The UI Message Loop handles sending the Exit message to other loops."
        n85 = event-data() -> ()  [unwired: 1 in, 1 out]
        n86 = call-poly "Enqueue Message.vi"("Priority Message? (F)"=w274, "Message"="Exit", "Message Queue"=w273) -> ("error out"=w276:errorcluster, "dup Message Queue"=w272:refnum<queue>)  [unwired: 7 in]
      }
      event "PRL Visible": Value Change {
        n87 = event-data() -> ("NewVal"=w277:bool)  [unwired: 1 in]
        n88 = Select(t=T20."Open Panel" ("Action"), s=w277, f=T20."Close Panel" ("Action")) -> (s? t:f=w283:T20)
        n89 = call <vilib>:"PRL Remote.vi"("error in (no error)"=w279, "Action"=w283) -> ("error out"=w278:errorcluster)  [unwired: 4 in, 5 out]
      }
      event "Data Selector": Value Change {
        n90 = event-data() -> ("NewVal"=w284:bool)  [unwired: 1 in]
        n91 = vi-ref "S3DK.lvlib:PMU Recorder Light.lvlib:PRL Channel Selector.vi"() -> (w288:refnum<vi>)
        n92 = case shown="False" w284 {
          tunnel: w288 -> [w291 w296]
          tunnel: w287 -> [w290 w292]
          tunnel: [w289 w293] -> w286
          frame False {
            n93 = invoke class="VI" method="FP.Close"(reference=w291, error in=w290) -> (error out=w289:errorcluster)  [unwired: 1 in, 2 out]
          }
          frame True {
            n94 = invoke class="VI" method="FP.Open"(reference=w296, error in=w292, "Activate"=TRUE ("Activate?"), "State"=T21."Standard") -> (error out=w293:errorcluster)  [unwired: 1 in, 4 out]
          }
        }
      }
      event User Event {
        # "The Message Handling Loop processed an \"Exit\" message, which fired this event to stop the Event Handling Loop."
        n95 = event-data() -> ()  [unwired: 1 in, 1 out]
        n96 = local write "Status"("Exit" ("Exit String")) -> ()
      }
    }
    n97 = call "Error Handler - Event Handling Loop.vi"("error in (no error)"=w244, "Message Queue"=w243) -> ("dup error in"=w245:errorcluster)  [unwired: 8 in, 1 out]
  }
  n98 = while {
    tunnel: w22 -> [w316]
    shift-right: [w312] -> _
    shift-left: w39 -> [w313]
    shift-right: [w309] -> _
    shift-left: w38 -> [w310]
    tunnel: w15 -> [w305]
    shift-right: [w306] -> _
    shift-left: _ -> [w307]
    tunnel: [w305] -> w27
    shift-right: [w304] -> w32
    shift-left: w35 -> [w300]
    stop <- w317 stop-if-true
    # "UI Message Loop"
    n99 = Not(x=w307) -> (.not. x?=w306:bool)
    "UI Control" <- w306
    n100 = Unbundle By Name(w305) -> ("UI"=w303:refnum<queue>)
    n101 = call "Error Handler - Message Handling Loop.vi"("error in (no error)"=w300, "Message Queue"=w303) -> ("dup error in"=w301:errorcluster, "dup Message Queue"=w302:refnum<queue>)  [unwired: 8 in]
    n102 = call "Dequeue Message.vi"("error in (no error)"=w301, "Message Queue"=w302) -> ("error out"=w308:errorcluster, "Message Data"=w314:variant, "Message"=w315:string, "dup Message Queue"=w311:refnum<queue>)  [unwired: 6 in]
    n103 = case "Message Cases" shown="\"Update Status (Acq)\"" w315 {
      selector: w315 -> [_ _ _ _ _ _ _ _ _ _ _ _ _ _ w599]
      tunnel: w311 -> [w319 _ _ _ _ w418 _ w440 w464 _ _ w556 _ _ _]
      tunnel: w308 -> [w320 w346 w353 w365 w394 w417 w420 w441 w465 w494 w545 w555 w585 w597 _]
      tunnel: [w327 w346 w354 w379 w393 w402 w435 w438 w462 w502 w548 w554 w591 w596 w598] -> w304
      tunnel: [_ _ _ _ _ _ _ _ _ _ _ _ TRUE _ _] -> w317
      tunnel: w314 -> [_ _ w352 _ _ _ _ _ _ _ w549 _ w587 _ _]
      tunnel: w316 -> [_ _ _ _ _ _ _ _ _ _ _ _ w592 _ _]
      tunnel: w313 -> [w324 w345 w348 w378 w396 w414 w434 w443 w467 w504 w552 w558 w590 w595 w601]
      tunnel: [w324 w332 w348 w378 w396 w414 w434 w443 w467 w504 w552 w558 w590 w595 w601] -> w312
      tunnel: w310 -> [_ _ w347 w377 w389 _ w424 w442 w466 w503 w547 w557 _ w594 w600]
      tunnel: [UI_State."Idle" ("UI State") UI_State."Idle" ("UI State") w347 w377 w389 UI_State."Acquiring and Logging" ("UI State") w425 w439 w463 w503 w547 w553 UI_State."Idle" ("UI State") w594 w600] -> w309
      tunnel: w305 -> [_ _ _ w369 w395 w397 w421 _ _ w501 _ _ w580 _ _]
      frame "Initialize" {
        # "Initialize - Get configuration settings, then message the UI to initialize, and broadcast the settings to the other message loops."
        n104 = call-poly "Enqueue Message.vi"("error in (no error)"=w320, "Message"="Init UI Refs", "Message Queue"=w319) -> ("error out"=w321:errorcluster, "dup Message Queue"=w322:refnum<queue>)  [unwired: 7 in]
        n105 = call-poly "Enqueue Message.vi"("error in (no error)"=w321, "Message Data"="Ready..." ("Ready..."), "Message"="Update Status", "Message Queue"=w322) -> ("error out"=w327:errorcluster)  [unwired: 6 in, 1 out]
      }
      frame "Init UI Refs" {
        # "Enable: Start, Exit, Settings \nDisable: Stop"
        # "Init UI Refs - Store control references for UI controls.  Also enable/disable controls appropriately."
        n106 = control-ref of="Data Selector"() -> (w334:refnum<vi>)
        n107 = control-ref of="PRL Visible"() -> (w333:refnum<vi>)
        n108 = control-ref of="Start"() -> (w338:refnum<vi>)
        n109 = control-ref of="Stop"() -> (w339:refnum<vi>)
        n110 = control-ref of="Settings"() -> (w337:refnum<vi>)
        n111 = control-ref of="Exit"() -> (w336:refnum<vi>)
        n112 = control-ref of="Status"() -> (w344:refnum<vi>)
        n113 = Bundle By Name(cluster=w345, "Start Ref"=w338, "Stop Ref"=w339, "Settings Ref"=w337, "Exit Ref"=w336, "Status Ref"=w344, "Data Selector"=w334, "PRL Visible"=w333) -> (w332:T14)
        n114 = Unbundle By Name(w332) -> ("Start Ref"=w331:refnum<vi>, "Exit Ref"=w330:refnum<vi>, "Settings Ref"=w329:refnum<vi>, "Stop Ref"=w328:refnum<vi>)
        n115 = Build Array(w331, w330, w329) -> (w342:refnum<vi>[])
        n116 = Build Array(w328) -> (w341:refnum<vi>[])
        n117 = call "Set Enable State on Multiple Controls.vi"("Enable?"=TRUE, "Controls"=w342) -> ()  [unwired: 10 in]
        n118 = call "Set Enable State on Multiple Controls.vi"("Enable?"=FALSE, "Controls"=w341) -> ()  [unwired: 10 in]
      }
      frame "Update Status" {
        # "Update Status - Convert the message data to a string to display in the Status indicator."
        n119 = Variant To Data(error in=w353, type="", Variant=w352) -> (data=→"Status":string, error out=w350:errorcluster)
        n120 = Merge Errors(w350) -> (w354:errorcluster)
      }
      frame "Update Status (Acq)" {
        # "Duplicate this frame when creating new messages.  Change this comment in the duplicated frame to describe this message."
        n121 = Obtain Queue(max queue size (-1, unlimited)=1, element data type=variant, error in (no error)=w365) -> (queue out=w362:refnum<queue>, error out=w380:errorcluster)  [unwired: 2 in, 1 out]
        n122 = Unbundle By Name(w369) -> ("Acquisition"=w364:refnum<queue>)
        n123 = Dequeue Element(queue=w362, timeout in ms (-1)=2000, error in (no error)=w380) -> (queue out=w366:refnum<queue>, element=w357:variant, error out=w367:errorcluster)  [unwired: 1 out]
        n124 = Release Queue(queue=w366, error in (no error)=w367) -> (error out=w356:errorcluster)  [unwired: 1 in, 2 out]
        n125 = call-poly "Enqueue Message.vi"("Priority Message? (F)"=TRUE, "error in (no error)"=w380, "Message Data"=w362, "Message"="Read Settings", "Message Queue"=w364) -> ("error out"=w363:errorcluster)  [unwired: 5 in, 1 out]
        n126 = Variant To Data(error in=w356, type=T9 {"State"=enum."Idle S3DK", "Settings"="Acquisition", "Online"=FALSE, "S3DK"={"Signals"={"Phasor"=[], "Analog"=[], "Digital"=[]}}, "CSV"={"Index"=0, "Parcel Length"=0, "EOF?"=FALSE, "Config"={"Mode"=enum."Full timestamp", "delimiter (\\t)"="\t", "Path"=path "", "Rectangular?"=FALSE}}} ("Acquisition Configuration"), Variant=w357) -> (data=w359:T9, error out=w355:errorcluster)
        n127 = Unbundle By Name(w359) -> ("Online"=w372:bool)
        n128 = call <vilib>:"Clear Errors.vi"("error in (no error)"=w355) -> ()  [unwired: 5 in, 2 out]
        n129 = case shown="False" w372 {
          tunnel: [w385 _] -> w376
          tunnel: [w384 _] -> w375
          tunnel: [w383 _] -> w374
          tunnel: [w381 _] -> w373
          frame True {
            n130 = call <vilib>:"PRL Remote.vi"("Action"=T20."Get Status") -> ("error out"=w382:errorcluster, "Connected"=w383:bool, "Configuration File Received"=w384:bool, "Buffer Active"=w387:bool, "Queue Active"=w386:bool)  [unwired: 5 in, 1 out]
            n131 = Unbundle By Name(w382) -> ("status"=w381:bool)
            n132 = Or(x=w386, y=w387) -> (x .or. y?=w385:bool)
          }
          frame False {
          }
        }
        "Buffer Active" <- w376
        "Config File" <- w375
        "Connected" <- w374
        "Error" <- w373
        n133 = Merge Errors(w363) -> (w379:errorcluster)
      }
      frame "Reset PSDs" {
        w390 = TRUE
        n134 = Unbundle By Name(w395) -> ("Processing"=w392:refnum<queue>)
        n135 = call-poly "Enqueue Message.vi"("Priority Message? (F)"=w390, "error in (no error)"=w394, "Message Data"=w390, "Message"="Process", "Message Queue"=w392) -> ("error out"=w393:errorcluster)  [unwired: 5 in, 1 out]
      }
      frame "Start" {
        # "Message Acquisition and Logging loops to start."
        # "Enable: Stop\nDisable: Start, Exit, Settings"
        # "Start - Enable/Disable buttons appropriately for an acquisition that has started, and update status display."
        n136 = Unbundle By Name(w414) -> ("Stop Ref"=w409:refnum<vi>, "Start Ref"=w408:refnum<vi>, "Exit Ref"=w407:refnum<vi>, "Settings Ref"=w406:refnum<vi>)
        n137 = call-poly "Enqueue Message.vi"("error in (no error)"=w417, "Message Data"="Acquiring and Logging..." ("Acquiring and Logging..."), "Message"="Update Status", "Message Queue"=w418) -> ("error out"=w405:errorcluster)  [unwired: 6 in, 1 out]
        n138 = Build Array(w408, w407, w406) -> (w412:refnum<vi>[])
        n139 = Build Array(w409) -> (w411:refnum<vi>[])
        n140 = Unbundle By Name(w397) -> ("Acquisition"=w398:refnum<queue>)
        n141 = call "Set Enable State on Multiple Controls.vi"("Enable?"=TRUE, "Controls"=w411) -> ()  [unwired: 10 in]
        n142 = call "Set Enable State on Multiple Controls.vi"("Enable?"=FALSE, "Controls"=w412) -> ()  [unwired: 10 in]
        n143 = call-poly "Enqueue Message.vi"("error in (no error)"=w405, "Message"="Start", "Message Queue"=w398) -> ("error out"=w403:errorcluster)  [unwired: 7 in, 1 out]
        n144 = Unbundle By Name(w397) -> ("Logging"=w399:refnum<queue>)
        n145 = call-poly "Enqueue Message.vi"("error in (no error)"=w403, "Message"="Start", "Message Queue"=w399) -> ("error out"=w402:errorcluster)  [unwired: 7 in, 1 out]
      }
      frame "Stop" {
        # "Message Acquisition, Logging and Process loops to stop"
        # "Enable: Start, Exit, Settings\nDisable: Stop"
        # "Stop - Enable/Disable buttons appropriately for an acquisition that has stopped, and update status display."
        n146 = call-poly "Enqueue Message.vi"("Exclude"="UI", "error in (no error)"=w420, "Message"="Stop", "Message Queues in"=w421) -> ("error out"=w422:errorcluster)  [unwired: 6 in, 1 out]
        n147 = Unbundle By Name(w434) -> ("Stop Ref"=w429:refnum<vi>, "Start Ref"=w428:refnum<vi>, "Exit Ref"=w427:refnum<vi>, "Settings Ref"=w426:refnum<vi>)
        n148 = Build Array(w428, w427, w426) -> (w432:refnum<vi>[])
        n149 = Build Array(w429) -> (w431:refnum<vi>[])
        n150 = call "Set Enable State on Multiple Controls.vi"("Enable?"=FALSE, "Controls"=w431) -> ()  [unwired: 10 in]
        n151 = call "Set Enable State on Multiple Controls.vi"("Enable?"=TRUE, "Controls"=w432) -> ()  [unwired: 10 in]
        n152 = case shown="Default" w424 {
          selector: w424 -> [w436 _]
          tunnel: [w436 UI_State."Waiting for Stop" ("UI State")] -> w425
          frame "Waiting for Exit" {
          }
          frame Default {
          }
        }
        n153 = Merge Errors(w422) -> (w435:errorcluster)
      }
      frame "Acquisition Stopped" {
        # "Logic for determining what action to take when the acquisition has stopped."
        n154 = case shown="\"Waiting for Stop (Log Stopped)\"" w442 {
          selector: w442 -> [w445 _ _ _ _]
          tunnel: w441 -> [w444 w447 w449 w455 w461]
          tunnel: w440 -> [_ _ _ w453 w458]
          tunnel: [w445 UI_State."Waiting for Exit (Acq Stopped)" ("UI State") UI_State."Waiting for Stop (Acq Stopped)" ("UI State") UI_State."Idle" ("UI State") UI_State."Idle" ("UI State")] -> w439
          tunnel: [w444 w447 w449 w454 w459] -> w438
          frame Default {
          }
          frame "Waiting for Exit", "Waiting for Exit (Acq Stopped)" {
          }
          frame "Waiting for Stop", "Waiting for Stop (Acq Stopped)" {
          }
          frame "Waiting for Exit (Log Stopped)" {
            # "If we are waiting to exit, and the logging has already stopped, then the \"Acquisition Stopped\" message indicates that it is time to exit."
            n155 = call-poly "Enqueue Message.vi"("Priority Message? (F)"=TRUE, "error in (no error)"=w455, "Message"="Exit", "Message Queue"=w453) -> ("error out"=w454:errorcluster)  [unwired: 6 in, 1 out]
          }
          frame "Waiting for Stop (Log Stopped)" {
            # "If we are waiting to stop, and the logging has already stopped, then the \"Acquisition Stopped\" message indicates that it is time to stop."
            n156 = call-poly "Enqueue Message.vi"("error in (no error)"=w461, "Message Data"="Ready..." ("Ready..."), "Message"="Update Status", "Message Queue"=w458) -> ("error out"=w459:errorcluster)  [unwired: 6 in, 1 out]
          }
        }
      }
      frame "Logging Stopped" {
        # "Logic for determining what action to take when the logging has stopped."
        n157 = case shown="\"Waiting for Exit (Acq Stopped)\"" w466 {
          selector: w466 -> [w469 _ _ _ _]
          tunnel: w465 -> [w468 w471 w473 w479 w482]
          tunnel: w464 -> [_ _ _ w477 w481]
          tunnel: [w469 UI_State."Waiting for Exit (Log Stopped)" ("UI State") UI_State."Waiting for Stop (Log Stopped)" ("UI State") UI_State."Idle" ("UI State") UI_State."Idle" ("UI State")] -> w463
          tunnel: [w468 w471 w473 w478 w480] -> w462
          frame Default {
          }
          frame "Waiting for Exit", "Waiting for Exit (Log Stopped)" {
          }
          frame "Waiting for Stop", "Waiting for Stop (Log Stopped)" {
          }
          frame "Waiting for Exit (Acq Stopped)" {
            # "If we are waiting to exit, and the acquisition has already stopped, then the \"Logging Stopped\" message indicates that it is time to exit."
            n158 = call-poly "Enqueue Message.vi"("Priority Message? (F)"=TRUE, "error in (no error)"=w479, "Message"="Exit", "Message Queue"=w477) -> ("error out"=w478:errorcluster)  [unwired: 6 in, 1 out]
          }
          frame "Waiting for Stop (Acq Stopped)" {
            # "If we are waiting to stop, and the acquisition has already stopped, then the \"Logging Stopped\" message indicates that it is time to stop."
            n159 = call-poly "Enqueue Message.vi"("error in (no error)"=w482, "Message Data"="Ready..." ("Ready..."), "Message"="Update Status", "Message Queue"=w481) -> ("error out"=w480:errorcluster)  [unwired: 6 in, 1 out]
          }
        }
      }
      frame "Launch Settings Dialog" {
        # "Launch Settings Dialog - Launch the Settings Dialog when the user clicks the 'Settings' button."
        n160 = for {
          N: 3 -> [_]
          tunnel: [w516] -> w493 mode=indexing
          tunnel: variant -> [w515]
          shift-right: [w513] -> w487
          shift-left: w494 -> [w514]
          n161 = Obtain Queue(max queue size (-1, unlimited)=1, element data type=w515, error in (no error)=w514) -> (queue out=w516:refnum<queue>, error out=w513:errorcluster)  [unwired: 2 in, 1 out]
        }
        n162 = call "Enqueue Message (same to all queues).vi"("Priority"=TRUE, "Exclude"="UI" ("y"), "error in (no error)"=w487, "Message Data Array"=w493, "Message"="Read Settings", "Message Queues in"=w501) -> ("error out"=w486:errorcluster, "Message Queues out"=w500:T15)  [unwired: 4 in]
        n163 = for {
          tunnel: w493 -> [w512] mode=indexing
          tunnel: [w511] -> w492 mode=indexing
          tunnel: [w508] -> w491 mode=indexing
          tunnel: 2000 ("timeout in ms (-1)") -> [w507]
          tunnel: [w506] -> w488
          tunnel: w486 -> [w505]
          n164 = Dequeue Element(queue=w512, timeout in ms (-1)=w507, error in (no error)=w505) -> (queue out=w509:refnum<queue>, element=w511:variant, timed out?=w508:bool, error out=w510:errorcluster)
          n165 = Release Queue(queue=w509, error in (no error)=w510) -> (error out=w506:errorcluster)  [unwired: 1 in, 2 out]
        }
        n166 = Or Array Elements(Boolean array=w491) -> (logical OR=w490:bool)
        n167 = call <vilib>:"Clear Errors.vi"("error in (no error)"=w488) -> ()  [unwired: 5 in, 2 out]
        n168 = case shown="False" w490 {
          tunnel: [w526 w543] -> w502
          tunnel: w486 -> [w521 w543]
          tunnel: w500 -> [w524 _]
          tunnel: w492 -> [w522 _]
          frame False {
            n169 = Array To Cluster(array=w522) -> (cluster=w523:T23)
            n170 = Variant To Data(error in=w521, type=T22 {"Acquisition"={"State"=enum."Idle S3DK", "Settings"="", "Online"=FALSE, "S3DK"={"Signals"={"Phasor"=[], "Analog"=[], "Digital"=[]}}, "CSV"={"Index"=0, "Parcel Length"=0, "EOF?"=FALSE, "Config"={"Mode"=enum."Full timestamp", "delimiter (\\t)"="\t", "Path"=path "", "Rectangular?"=FALSE}}}, "Logging"={"Logging State"=enum."Idle", "Settings"="", "Buffer"={"Index"=0, "Size"=15000, "Samples"=0, "Ordered ?"=FALSE}}, "Processing"={"Settings"="", "Parameters"={"Index"=0, "Size"=0, "Samples"=0, "Ordered ?"=FALSE}, "Refresh Rate"=0}} ("Settings in"), Variant=w523) -> (data=w519:T22, error out=w520:errorcluster)
            n171 = call-by-ref "?"("error in (no error)"=w520, "Settings in"=w519) -> ("error out"=w527:errorcluster, "Changed?"=w528:bool, "Settings out"=w525:T22)  [unwired: 8 in, 3 out]
            n172 = case shown="True" w528 {
              tunnel: w527 -> [w529 w536]
              tunnel: [w529 w535] -> w526
              tunnel: w525 -> [_ w530]
              tunnel: w524 -> [_ w532]
              frame False {
              }
              frame True {
                n173 = Unbundle(w530) -> ("Acquisition"=w542:T9, "Logging"=w541:T7, "Processing"=w540:T5)
                n174 = To Variant(anything=w542) -> (Variant=w539:variant)
                n175 = To Variant(anything=w541) -> (Variant=w538:variant)
                n176 = To Variant(anything=w540) -> (Variant=w537:variant)
                n177 = Build Array(w539, w538, w537) -> (w534:variant[])
                n178 = call "Enqueue Message (same to all queues).vi"("Exclude"="UI" ("y"), "error in (no error)"=w536, "Message Data Array"=w534, "Message"="Update Settings", "Message Queues in"=w532) -> ("error out"=w535:errorcluster)  [unwired: 5 in, 1 out]
              }
            }
          }
          frame True {
          }
        }
      }
      frame "Error" {
        w544 = T17 2 items=["no dialog", "OK message", "continue or stop message", "OK message + warnings", "continue/stop + warnings"] ("type of dialog (OK msg:1)")
        # "Error - Display an error dialog. This message is sent by the \"Error Handler\" VIs at the end of other loops in this application."
        n179 = Variant To Data(error in=w545, type=errorcluster {"status"=FALSE, "code"=0, "source"=""} ("error constant"), Variant=w549) -> (data=w546:errorcluster, error out=w550:errorcluster)
        n180 = call <vilib>:"Simple Error Handler.vi"("type of dialog (OK msg:1)"=w544, "error in (no error)"=w546) -> ()  [unwired: 3 in, 5 out]
        n181 = Merge Errors(w550) -> (w548:errorcluster)
      }
      frame "Confirm Quit" {
        # "Confirm Quit - Message that can confirm whether or not the user wants to exit the application."
        n182 = case shown="\"Acquiring and Logging\"" w557 {
          tunnel: w556 -> [w564 w568]
          tunnel: w555 -> [w563 w567]
          tunnel: [w562 w566] -> w554
          tunnel: [UI_State."Idle" ("UI State") w565] -> w553
          frame Default {
            # "If 'Confirm Quit' comes in while the system is idle, there is no need for a confirmation message."
            n183 = call-poly "Enqueue Message.vi"("Priority Message? (F)"=TRUE, "error in (no error)"=w563, "Message"="Exit", "Message Queue"=w564) -> ("error out"=w562:errorcluster)  [unwired: 6 in, 1 out]
          }
          frame "Acquiring and Logging" {
            n184 = Two Button Dialog(message="Are you sure you want to quit while the acquisition is running?" ("Confirm Quit Message"), 1:"No" ("No"), 2:"Yes" ("Yes")) -> (T button?=w569:bool)
            n185 = case shown="False" w569 {
              tunnel: w568 -> [_ w578]
              tunnel: w567 -> [w574 w579]
              tunnel: [w574 w577] -> w566
              tunnel: [UI_State."Acquiring and Logging" ("UI State") UI_State."Waiting for Exit" ("UI State")] -> w565
              frame False {
                # "User did not want to quit."
              }
              frame True {
                n186 = call-poly "Enqueue Message.vi"("error in (no error)"=w579, "Message"="Stop", "Message Queue"=w578) -> ("error out"=w577:errorcluster)  [unwired: 7 in, 1 out]
              }
            }
          }
        }
      }
      frame "Exit" {
        # "Popup an error dialog if 'Exit' was called as a result of an error."
        # "Stop the VI"
        # "Exit - Send Exit messages to the Acquisition and Logging loops, and fire the user event to stop the Event Handling Loop."
        n187 = Variant To Data(type=errorcluster {"status"=FALSE, "code"=0, "source"=""} ("error constant"), Variant=w587) -> (data=w586:errorcluster)  [unwired: 1 in, 1 out]
        n188 = call <vilib>:"Simple Error Handler.vi"("error in (no error)"=w586) -> ()  [unwired: 4 in, 5 out]
        n189 = call-poly "Enqueue Message.vi"("Priority"=TRUE ("Priority Message? (F)"), "Exclude"="UI", "error in (no error)"=w585, "Message"="Exit", "Message Queues in"=w580) -> ("error out"=w584:errorcluster)  [unwired: 5 in, 1 out]
        n190 = call "Fire User Event - Stop.vi"("error in (no error)"=w584, "User Event - Stop"=w592) -> ("error out"=w591:errorcluster)  [unwired: 9 in]
      }
      frame "---Copy This Frame---" {
        # "Duplicate this frame when creating new messages.  Change this comment in the duplicated frame to describe this message."
        n191 = Merge Errors(w597) -> (w596:errorcluster)
      }
      frame Default {
        # "'Default' case only runs if there is a message that isn't defined in any of the other cases.  Output a programming error."
        n192 = xnode "Error Ring"("parameter 0"=w599) -> ("error out"=w598:errorcluster)
      }
    }
  }
  n193 = while {
    shift-right: [w629] -> _
    shift-left: w14 -> [w617]
    tunnel: w34 -> [w624]
    tunnel: w15 -> [w622]
    shift-right: [w618] -> _
    shift-left: _ -> [w619]
    shift-right: [w614] -> w26
    shift-left: w16 -> [w612]
    tunnel: enum16{"OGnE", "WAN-OGE"}."OGnE" ("Original CSV Format") -> [w610]
    tunnel: w3 -> [w609]
    stop <- w628 stop-if-true
    # "Acquisition Loop"
    n194 = Unbundle By Name(w622) -> ("Logging"=w615:refnum<queue>, "UI"=w621:refnum<queue>, "Acquisition"=w620:refnum<queue>, "UI"=w611:refnum<queue>)
    n195 = Not(x=w619) -> (.not. x?=w618:bool)
    "Acquisition" <- w618
    n196 = Unbundle By Name(w617) -> ("State"=w616:T10)
    n197 = call "Error Handler - Acquisition Message Loop.vi"("error in (no error)"=w612, "Message Queue"=w611) -> ("dup error in"=w613:errorcluster)  [unwired: 8 in, 1 out]
    n198 = call "Dequeue Message.vi"("error in (no error)"=w613, "Message Queue"=w620) -> ("error out"=w627:errorcluster, "Message Data"=w625:variant, "Message"=w626:string, "dup Message Queue"=w623:refnum<queue>)  [unwired: 6 in]
    n199 = case "Message Cases" shown="\"Start\"" w626 {
      selector: w626 -> [_ _ w698 _ _ _ _ _ _ w865]
      tunnel: w623 -> [_ w649 w702 _ _ w770 _ _ _ _]
      tunnel: w627 -> [w637 w650 w701 w739 w760 w769 w806 w848 w864 _]
      tunnel: [w630 w651 w694 w740 w759 w766 w813 w852 w862 w866] -> w614
      tunnel: w617 -> [w636 w644 w696 w737 w762 w771 w811 w850 w863 w867]
      tunnel: [w632 w648 w695 w734 w762 w768 w810 w845 w863 w867] -> w629
      tunnel: [_ _ _ _ _ _ _ TRUE _ _] -> w628
      tunnel: w625 -> [_ _ _ _ w761 w774 _ _ _ _]
      tunnel: w621 -> [_ _ w693 w735 _ _ w809 _ _ _]
      tunnel: w624 -> [_ _ w700 _ _ _ _ _ _ _]
      tunnel: w616 -> [_ w647 w699 w736 _ _ w812 w846 _ _]
      tunnel: w615 -> [_ _ _ _ _ _ w808 _ _ _]
      tunnel: w610 -> [_ w642 _ _ _ _ _ _ _ _]
      tunnel: w609 -> [_ w641 _ _ _ _ _ _ _ _]
      frame "Initialize" {
        w638 = T17 2 items=["no dialog", "OK message", "continue or stop message", "OK message + warnings", "continue/stop + warnings"] ("type of dialog (OK msg:1)")
        # "Initialize  - Initialize is currently a no-op.  The hardware initialization takes place in the 'Start' message."
        n200 = Unbundle By Name(w636) -> ("Settings"=w631:string)
        n201 = call "Load Settings from XML.vim"("error in (no error)"=w637, "Settings File Name"=w631, "Settings In"=w636) -> ("error out"=w634:errorcluster, "Settings Out"=w633:T9)  [unwired: 7 in]
        n202 = Bundle By Name(cluster=w633, "State"=Acquisition_State."Idle" ("Acquisition State"), "Settings"=w631, "Online"=FALSE ("Status.Online")) -> (w632:T9)
        n203 = call <vilib>:"General Error Handler.vi"("[error source] (\" \")"="Acq. Settings" ("[error source] (\" \")"), "type of dialog (OK msg:1)"=w638, "error in (no error)"=w634) -> ("error out"=w630:errorcluster)  [unwired: 8 in, 4 out]
      }
      frame "Start" {
        # "Start - Configure and start the acquisition."
        n204 = Unbundle By Name(w644) -> ("Online"=w643:bool)
        n205 = call-poly "Enqueue Message.vi"("error in (no error)"=w650, "Message"="Acquire", "Message Queue"=w649) -> ("error out"=w645:errorcluster)  [unwired: 7 in, 1 out]
        n206 = case shown="\"Idle\"" w647 {
          tunnel: [w655 w660 w662 w667] -> w651
          tunnel: w644 -> [w657 w661 w663 w670]
          tunnel: [w653 w659 w663 w669] -> w648
          tunnel: w645 -> [w656 w660 w662 w666]
          tunnel: w643 -> [_ _ _ w668]
          tunnel: w642 -> [_ _ _ w665]
          tunnel: w641 -> [_ _ _ w664]
          frame "Idle S3DK" {
            # "Restart the PDC streaming real time data"
            n207 = call <vilib>:"PRL Remote.vi"("error in (no error)"=w656, "Action"=T20."Continue") -> ("error out"=w655:errorcluster)  [unwired: 4 in, 5 out]
            n208 = Bundle By Name(cluster=w657, "State"=Acquisition_State."Acquiring S3DK") -> (w653:T9)
          }
          frame "Idle CSV" {
            n209 = Bundle By Name(cluster=w661, "State"=Acquisition_State."Acquiring CSV") -> (w659:T9)
          }
          frame Default {
            # "By default, ignorre the message as not in IDLE state"
          }
          frame "Idle" {
            # "If the system is idle, start the acquisition."
            n210 = case shown="False" w668 {
              tunnel: w670 -> [w678 w689]
              tunnel: [w684 w691] -> w669
              tunnel: [w679 w686] -> w667
              tunnel: w666 -> [w675 w685]
              tunnel: w665 -> [w671 _]
              tunnel: w664 -> [w672 _]
              frame False {
                n211 = Unbundle By Name(w678) -> ("CSV.Config.Path"=w677:path, "CSV.Config.delimiter (\\t)"=w676:string)
                n212 = call "Format CSV.vi"("error in (no error)"=w675, "delimiter"=w676, "CSV File Input"=w677, "Original CSV Format"=w671) -> ("error out"=w674:errorcluster, "All Terminal Data"=w673:T24[])  [unwired: 5 in, 1 out]
                n213 = call "Configure CSV.vi"("Original CSV Format"=w671, "error in (no error)"=w674, "Run Mode Est Settings"=w672, "All Terminal Data"=w673, "Settings IN"=w678) -> ("error out"=w680:errorcluster, "Settings OUT"=w682:T9)  [unwired: 4 in, 1 out]
                n214 = call "Initialize CSV.vi"("error in (no error)"=w680, "Settings IN"=w682) -> ("error out"=w679:errorcluster, "Settings OUT"=w681:T9)  [unwired: 8 in]
                n215 = Bundle By Name(cluster=w681, "State"=Acquisition_State."Acquiring CSV") -> (w684:T9)
              }
              frame True {
                n216 = call "Initialize S3DK.vi"("error in (no error)"=w685, "Settings IN"=w689) -> ("error out"=w688:errorcluster, "Settings OUT"=w687:T9)  [unwired: 8 in]
                n217 = call "Configure S3DK.vi"("error in (no error)"=w688, "Settings IN"=w687) -> ("error out"=w686:errorcluster, "Settings OUT"=w692:T9)  [unwired: 8 in]
                n218 = Bundle By Name(cluster=w692, "State"=Acquisition_State."Acquiring S3DK" ("Acquisition State")) -> (w691:T9)
              }
            }
          }
        }
      }
      frame "Acquire" {
        # "Throttling to a min of 10 ms in the loop"
        # "Acquire - Acquire data from the hardware. Since this is a continuous acquisition, this message will always message itself to run again."
        n219 = case shown="\"Acquiring CSV\"" w699 {
          tunnel: [w706 w712 w717] -> w694
          tunnel: w702 -> [w710 _ w720]
          tunnel: w701 -> [w709 w712 w721]
          tunnel: [w703 w711 w713] -> w695
          tunnel: w696 -> [w705 w711 w723]
          tunnel: w700 -> [w704 _ w724]
          tunnel: w698 -> [w708 _ w719]
          tunnel: w693 -> [_ _ w716]
          frame "Acquiring S3DK" {
            # "Acquire more data while in the \"Acquiring\" state."
            n220 = call-poly "Enqueue Message.vi"("error in (no error)"=w709, "Message"=w708, "Message Queue"=w710) -> ("error out"=w707:errorcluster)  [unwired: 7 in, 1 out]
            n221 = call "Acquire S3DK.vi"("error in (no error)"=w707, "DATA IN"=w704, "Hardware Resources in"=w705) -> ("error out"=w706:errorcluster, "Hardware Resources out"=w703:T9)  [unwired: 7 in]
          }
          frame Default {
          }
          frame "Acquiring CSV" {
            n222 = call-poly "Enqueue Message.vi"("error in (no error)"=w721, "Message"=w719, "Message Queue"=w720) -> ("error out"=w722:errorcluster)  [unwired: 7 in, 1 out]
            n223 = call "Acquire CSV.vi"("error in (no error)"=w722, "DATA IN"=w724, "Hardware Resources in"=w723) -> ("error out"=w718:errorcluster, "Hardware Resources out"=w714:T9)  [unwired: 7 in]
            n224 = Unbundle By Name(w714) -> ("CSV.EOF?"=w715:bool)
            n225 = case shown="False" w715 {
              tunnel: w718 -> [w726 w732]
              tunnel: [w726 w731] -> w717
              tunnel: w716 -> [_ w730]
              tunnel: w714 -> [w725 w729]
              tunnel: [w725 w728] -> w713
              frame False {
              }
              frame True {
                n226 = Bundle By Name(cluster=w729, "CSV.Index"=0 ("CSV .Index (file reading)")) -> (w728:T9)
                n227 = call-poly "Enqueue Message.vi"("error in (no error)"=w732, "Message"="Stop", "Message Queue"=w730) -> ("error out"=w731:errorcluster)  [unwired: 7 in, 1 out]
              }
            }
          }
        }
        n228 = Wait Until Next ms Multiple(millisecond multiple=u32 10) -> ()  [unwired: 1 out]
      }
      frame "Stop" {
        # "Stop - Stop the Acquisition."
        n229 = case shown="\"Acquiring CSV\"" w736 {
          tunnel: w739 -> [w742 w748 w754]
          tunnel: [w742 w743 w751] -> w738
          tunnel: w737 -> [w741 w747 w753]
          tunnel: w735 -> [_ w750 w755]
          tunnel: [w741 w746 w757] -> w734
          frame Default {
            # "The system is already idle. Ignore the \"Stop\" message."
          }
          frame "Acquiring S3DK" {
            # "If the system is acquiring, stop the acquisition."
            n230 = call-poly "Enqueue Message.vi"("error in (no error)"=w748, "Message"="Acquisition Stopped", "Message Queue"=w750) -> ("error out"=w744:errorcluster)  [unwired: 7 in, 1 out]
            n231 = call "Stop S3DK.vi"("error in (no error)"=w744, "Hardware Resources in"=w747) -> ("error out"=w743:errorcluster)  [unwired: 9 in]
            n232 = Bundle By Name(cluster=w747, "State"=Acquisition_State."Idle S3DK") -> (w746:T9)
          }
          frame "Acquiring CSV" {
            n233 = call-poly "Enqueue Message.vi"("error in (no error)"=w754, "Message"="Acquisition Stopped", "Message Queue"=w755) -> ("error out"=w752:errorcluster)  [unwired: 7 in, 1 out]
            n234 = call "Stop CSV.vi"("error in (no error)"=w752, "Hardware Resources in"=w753) -> ("error out"=w751:errorcluster)  [unwired: 9 in]
            n235 = Bundle By Name(cluster=w753, "State"=Acquisition_State."Idle CSV") -> (w757:T9)
          }
        }
        n236 = Merge Errors(w738) -> (w740:errorcluster)
      }
      frame "Read Settings" {
        n237 = Variant To Data(error in=w760, type=refnum<queue> refnum ("queue out"), Variant=w761) -> (data=w763:refnum<queue>, error out=w764:errorcluster)
        n238 = Lossy Enqueue Element(queue=w763, element=w762, error in (no error)=w764) -> (error out=w759:errorcluster)  [unwired: 3 out]
      }
      frame "Update Settings" {
        # "New settings are available, update the current ones stored in the shift register with the settings sent as part of the message"
        n239 = Variant To Data(error in=w769, type=w771, Variant=w774) -> (data=w772:T9, error out=w773:errorcluster)
        n240 = Select(t=w771, s=w773, f=w772) -> (s? t:f=w767:T9)
        n241 = stacked-sequence {
          tunnel: w767 -> [w779 w793]
          tunnel: w771 -> [w780 w794]
          tunnel: w770 -> [w777 _]
          tunnel: w769 -> [w776 _]
          tunnel: w767 -> [_ w791]
          tunnel: [_ w790] -> w768
          tunnel: w767 -> [_ w788]
          tunnel: [w775 _] -> w766
          frame #0 {
            n242 = Unbundle By Name(w780) -> ("Online"=w781:bool)
            n243 = Unbundle By Name(w779) -> ("Online"=w782:bool)
            n244 = Not Equal?(x=w781, y=w782) -> (x != y?=w778:bool)
            n245 = case shown="True" w778 {
              tunnel: w776 -> [w783 w787]
              tunnel: [w783 w786] -> w775
              tunnel: w777 -> [_ w785]
              frame False {
              }
              frame True {
                # "Change Data source"
                n246 = call-poly "Enqueue Message.vi"("error in (no error)"=w787, "Message"="Toggle Online", "Message Queue"=w785) -> ("error out"=w786:errorcluster)  [unwired: 7 in, 1 out]
              }
            }
          }
          frame #1 {
            n247 = Unbundle By Name(w794) -> ("CSV.Config.Path"=w795:path)
            n248 = Unbundle By Name(w793) -> ("CSV.Config.Path"=w796:path)
            n249 = Not Equal?(x=w795, y=w796) -> (x != y?=w792:bool)
            n250 = case shown="True" w792 {
              tunnel: [w798 Acquisition_State."Idle" ("State")] -> w789
              tunnel: w788 -> [w797 _]
              frame False {
                n251 = Unbundle By Name(w797) -> ("State"=w798:T10)
              }
              frame True {
              }
            }
            n252 = Bundle By Name(cluster=w791, "State"=w789) -> (w790:T9)
          }
        }
      }
      frame "Toggle Online" {
        # "Duplicate this frame when creating new messages.  Change this comment in the duplicated frame to describe this message."
        n253 = call-poly "Enqueue Message.vi"("error in (no error)"=w806, "Message"="Flush", "Message Queue"=w808) -> ("error out"=w805:errorcluster)  [unwired: 7 in, 1 out]
        n254 = case shown="\"Idle S3DK\", \"Acquiring S3DK\"" w812 {
          tunnel: w811 -> [w820 w831 w840]
          tunnel: [w820 w822 w834] -> w810
          tunnel: [w817 w826 w837] -> w801
          tunnel: w805 -> [w818 w830 w841]
          tunnel: w809 -> [w815 w829 w842]
          tunnel: [w814 w823 w835] -> w800
          frame "Idle", Default {
            n255 = call-poly "Enqueue Message.vi"("error in (no error)"=w818, "Message Data"="Toggle Data source" ("Message"), "Message"="Update Status", "Message Queue"=w815) -> ("error out"=w817:errorcluster, "dup Message Queue"=w814:refnum<queue>)  [unwired: 6 in]
          }
          frame "Idle S3DK", "Acquiring S3DK" {
            n256 = call-poly "Enqueue Message.vi"("error in (no error)"=w830, "Message Data"="Stopping the S3DK data acquisition" ("Ready..."), "Message"="Update Status", "Message Queue"=w829) -> ("error out"=w824:errorcluster, "dup Message Queue"=w823:refnum<queue>)  [unwired: 6 in]
            n257 = Bundle By Name(cluster=w831, "State"=Acquisition_State."Idle") -> (w822:T9)
            n258 = call "Stop S3DK.vi"("error in (no error)"=w824, "Hardware Resources in"=w822) -> ("error out"=w832:errorcluster)  [unwired: 9 in]
            n259 = call "Shutdown S3DK.vi"("error in (no error)"=w832, "Hardware Resources in"=w822) -> ("error out"=w825:errorcluster)  [unwired: 9 in]
            n260 = Merge Errors(w825, w824) -> (w826:errorcluster)
          }
          frame "Idle CSV", "Acquiring CSV" {
            n261 = call-poly "Enqueue Message.vi"("error in (no error)"=w841, "Message Data"="Stopping the CSV data acquisition" ("Ready..."), "Message"="Update Status", "Message Queue"=w842) -> ("error out"=w836:errorcluster, "dup Message Queue"=w835:refnum<queue>)  [unwired: 6 in]
            n262 = Bundle By Name(cluster=w840, "State"=Acquisition_State."Idle") -> (w834:T9)
            n263 = call "Stop CSV.vi"("error in (no error)"=w836, "Hardware Resources in"=w834) -> ("error out"=w839:errorcluster)  [unwired: 9 in]
            n264 = call "Shutdown CSV.vi"("error in (no error)"=w839, "Hardware Resources in"=w834) -> ("error out"=w838:errorcluster)  [unwired: 9 in]
            n265 = Merge Errors(w838, w836) -> (w837:errorcluster)
          }
        }
        n266 = call-poly "Enqueue Message.vi"("error in (no error)"=w801, "Message Data"="Ready..." ("Ready..."), "Message"="Update Status", "Message Queue"=w800) -> ("error out"=w802:errorcluster)  [unwired: 6 in, 1 out]
        n267 = Merge Errors(w802) -> (w813:errorcluster)
      }
      frame "Exit" {
        # "Stop the VI"
        # "Exit - Send the Exit message to the UI Message Handler."
        n268 = case shown="\"Idle CSV\", \"Acquiring CSV\"" w846 {
          tunnel: w850 -> [w854 w856 w859]
          tunnel: [w855 w857 w861] -> w849
          tunnel: w848 -> [w855 w858 w860]
          tunnel: [w854 w856 w859] -> w845
          frame "Idle", Default {
          }
          frame "Idle CSV", "Acquiring CSV" {
            n269 = call "Shutdown CSV.vi"("error in (no error)"=w858, "Hardware Resources in"=w856) -> ("error out"=w857:errorcluster)  [unwired: 9 in]
          }
          frame "Idle S3DK", "Acquiring S3DK" {
            n270 = call "Shutdown S3DK.vi"("error in (no error)"=w860, "Hardware Resources in"=w859) -> ("error out"=w861:errorcluster)  [unwired: 9 in]
          }
        }
        n271 = Unbundle By Name(w845) -> ("Settings"=w851:string)
        n272 = call "Save Settings to XML.vim"("error in (no error)"=w849, "Settings File Name"=w851, "Settings In"=w845) -> ("error out"=w847:errorcluster)  [unwired: 8 in]
        n273 = Merge Errors(w847) -> (w852:errorcluster)
      }
      frame "---Copy This Frame---" {
        # "Duplicate this frame when creating new messages.  Change this comment in the duplicated frame to describe this message."
        n274 = Merge Errors(w864) -> (w862:errorcluster)
      }
      frame Default {
        # "'Default' case only runs if there is a message that isn't defined in any of the other cases.  Output a programming error."
        n275 = xnode "Error Ring"("parameter 0"=w865) -> ("error out"=w866:errorcluster)
      }
    }
  }
  n276 = while {
    shift-right: [w882] -> _
    shift-left: w12 -> [w884]
    tunnel: w34 -> [w881]
    tunnel: w15 -> [w880]
    shift-right: [w885] -> _
    shift-left: _ -> [w886]
    tunnel: [w881] -> w28
    shift-right: [w878] -> w25
    shift-left: w16 -> [w876]
    stop <- w893 stop-if-true
    # "Logging Loop"
    n277 = Unbundle By Name(w880) -> ("Processing"=w879:refnum<queue>, "UI"=w887:refnum<queue>, "Logging"=w888:refnum<queue>, "UI"=w875:refnum<queue>)
    n278 = Unbundle By Name(w884) -> ("Logging State"=w883:T8)
    n279 = Not(x=w886) -> (.not. x?=w885:bool)
    "Buffer" <- w885
    n280 = call "Error Handler - Logging Message Loop.vi"("error in (no error)"=w876, "Message Queue"=w875) -> ("dup error in"=w877:errorcluster)  [unwired: 8 in, 1 out]
    n281 = call "Dequeue Message.vi"("error in (no error)"=w877, "Message Queue"=w888) -> ("error out"=w892:errorcluster, "Message Data"=w890:variant, "Message"=w891:string, "dup Message Queue"=w889:refnum<queue>)  [unwired: 6 in]
    n282 = case "Message Cases" shown="\"Log\"" w891 {
      selector: w891 -> [_ w909 _ _ _ _ _ _ _ w1017]
      tunnel: w889 -> [_ w914 w930 _ _ _ _ _ _ _]
      tunnel: w892 -> [w902 w908 w928 w958 w987 w989 w1006 w1012 w1016 _]
      tunnel: [w894 w915 w931 w961 w981 w999 w1008 w1011 w1014 w1018] -> w878
      tunnel: w884 -> [w903 w913 w927 w955 w982 w997 w1003 w1013 w1015 w1019]
      tunnel: [w896 w912 w927 w954 w982 w994 w1003 w1013 w1015 w1019] -> w882
      tunnel: [_ _ _ _ _ _ TRUE _ _ _] -> w893
      tunnel: w890 -> [_ _ _ _ w986 w998 _ _ _ _]
      tunnel: w887 -> [_ _ _ w956 _ _ _ _ _ _]
      tunnel: w881 -> [_ _ w929 w959 _ _ w1007 _ _ _]
      tunnel: w883 -> [_ w911 w926 w957 _ w993 _ _ _ _]
      tunnel: w879 -> [_ w910 _ _ _ _ _ _ _ _]
      frame "Initialize" {
        w905 = T17 2 items=["no dialog", "OK message", "continue or stop message", "OK message + warnings", "continue/stop + warnings"] ("type of dialog (OK msg:1)")
        # "Initialize - gets called when first launched. Currently a no-op."
        n283 = Unbundle By Name(w903) -> ("Settings"=w895:string)
        n284 = call "Load Settings from XML.vim"("error in (no error)"=w902, "Settings File Name"=w895, "Settings In"=w903) -> ("error out"=w898:errorcluster, "Settings Out"=w897:T7)  [unwired: 7 in]
        n285 = Bundle By Name(cluster=w897, "Logging State"=Logging_State."Idle" ("State"), "Settings"=w895) -> (w896:T7)
        n286 = Unbundle By Name(w896) -> ("Buffer"=w900:T6)
        n287 = call "Buffer.vi"("Parameters"=w900, "Mode"=Buffer_state."Init", "Error IN"=w898) -> ("Error OUT"=w899:errorcluster)  [unwired: 4 in, 4 out]
        n288 = call <vilib>:"General Error Handler.vi"("[error source] (\" \")"="Log. Settings" ("[error source] (\" \")"), "type of dialog (OK msg:1)"=w905, "error in (no error)"=w899) -> ("error out"=w894:errorcluster)  [unwired: 8 in, 4 out]
      }
      frame "Start" {
        # "Start - Send the \"Log\" message to start logging.  Generate a unique, timestamped TDMS file name based on the Log File Base Path value."
        n289 = call-poly "Enqueue Message.vi"("error in (no error)"=w908, "Message"=w909, "Message Queue"=w910) -> ("error out"=w907:errorcluster)  [unwired: 7 in, 1 out]
        n290 = case shown="\"Idle\"" w911 {
          tunnel: [w916 w921] -> w915
          tunnel: w914 -> [_ w922]
          tunnel: w907 -> [w916 w920]
          tunnel: w913 -> [w917 w923]
          tunnel: [w917 w924] -> w912
          frame "Logging" {
            # "The system is already logging. Ignore the \"Start\" message."
          }
          frame "Idle" {
            # "If the system is idle, start logging."
            n291 = call-poly "Enqueue Message.vi"("error in (no error)"=w920, "Message"="Log", "Message Queue"=w922) -> ("error out"=w918:errorcluster)  [unwired: 7 in, 1 out]
            n292 = Bundle By Name(cluster=w923, "Logging State"=Logging_State."Logging" ("State")) -> (w924:T7)
            n293 = Merge Errors(w918) -> (w921:errorcluster)
          }
        }
      }
      frame "Log" {
        # "Log - Log data to disk. Since this is a continuous acquisition, this message will always message itself to run again."
        n294 = case shown="\"Logging\"" w926 {
          tunnel: [w932 w944] -> w931
          tunnel: w930 -> [_ w943]
          tunnel: w929 -> [_ w939]
          tunnel: w928 -> [w932 w941]
          frame "Idle" {
            # "Ignore \"Log\" messages when the logging is idle."
          }
          frame "Logging" {
            # "Throttling to a minimum\nof 15 ms in loop"
            # "Log more data while in the \"Logging\" state."
            n295 = call-poly "Enqueue Message.vi"("error in (no error)"=w941, "Message"="Log", "Message Queue"=w943) -> ("error out"=w934:errorcluster)  [unwired: 7 in, 1 out]
            n296 = Flush Queue(queue=w939, error in (no error)=w934) -> (remaining elements=w938:cluster{T13[]}[], error out=w935:errorcluster)  [unwired: 1 out]
            n297 = for {
              tunnel: w938 -> [w946] mode=indexing
              tunnel: [w945] -> w936 mode=concatenating
              n298 = Unbundle(w946) -> (w945:T13[])
            }
            n299 = Empty Array?(array=w936) -> (empty?=w937:bool)
            n300 = case shown="False" w937 {
              tunnel: w935 -> [w950 w953]
              tunnel: w936 -> [w951 _]
              tunnel: [w948 w953] -> w940
              tunnel: [u32 15 ("millisecond multiple") u32 100 ("millisecond multiple")] -> w933
              frame False {
                n301 = call "Buffer.vi"("Mode"=Buffer_state."Add", "Error IN"=w950, "DATA IN"=w951) -> ("Error OUT"=w948:errorcluster)  [unwired: 4 in, 4 out]
              }
              frame True {
              }
            }
            n302 = Merge Errors(w940, w934) -> (w944:errorcluster)
            n303 = Wait Until Next ms Multiple(millisecond multiple=w933) -> ()  [unwired: 1 out]
          }
        }
      }
      frame "Stop" {
        # "Stop - Flush the message queue of any pending \"Log\" messages. Call 'Flush Data to Log File.vi' so any pending data is not lost."
        n304 = case shown="\"Logging\"" w957 {
          tunnel: [w963 w975] -> w960
          tunnel: w959 -> [_ w968]
          tunnel: w958 -> [w963 w969]
          tunnel: w956 -> [_ w974]
          tunnel: w955 -> [w962 w970]
          tunnel: [w962 w972] -> w954
          frame "Idle" {
            # "The system is already idle. Ignore the \"Stop\"."
          }
          frame "Logging" {
            # "If the system is logging, stop logging."
            n305 = Flush Queue(queue=w968, error in (no error)=w969) -> (remaining elements=w967:cluster{T13[]}[], error out=w966:errorcluster)  [unwired: 1 out]
            n306 = for {
              tunnel: w967 -> [w980] mode=indexing
              shift-right: [w978] -> w964
              shift-left: w966 -> [w977]
              tunnel: Buffer_state."Add" ("Mode") -> [w976]
              n307 = Unbundle(w980) -> (w979:T13[])
              n308 = call "Buffer.vi"("Mode"=w976, "Error IN"=w977, "DATA IN"=w979) -> ("Error OUT"=w978:errorcluster)  [unwired: 4 in, 4 out]
            }
            n309 = Bundle By Name(cluster=w970, "Logging State"=Logging_State."Idle" ("State")) -> (w972:T7)
            n310 = call-poly "Enqueue Message.vi"("error in (no error)"=w964, "Message"="Logging Stopped", "Message Queue"=w974) -> ("error out"=w975:errorcluster)  [unwired: 7 in, 1 out]
          }
        }
        n311 = Merge Errors(w960) -> (w961:errorcluster)
      }
      frame "Read Settings" {
        n312 = Variant To Data(error in=w987, type=refnum<queue> refnum ("queue out"), Variant=w986) -> (data=w983:refnum<queue>, error out=w984:errorcluster)
        n313 = Lossy Enqueue Element(queue=w983, element=w982, error in (no error)=w984) -> (error out=w981:errorcluster)  [unwired: 3 out]
      }
      frame "Update Settings" {
        # "Update Settings - New settings are available, update the current ones stored in the shift register with the settings sent as part of the message."
        n314 = Variant To Data(error in=w989, type=w997, Variant=w998) -> (data=w996:T7, error out=w995:errorcluster)
        n315 = Select(t=w997, s=w995, f=w996) -> (s? t:f=w992:T7)
        n316 = Unbundle By Name(w992) -> ("Buffer"=w991:T6)
        n317 = Bundle By Name(cluster=w992, "Logging State"=w993) -> (w994:T7)
        n318 = call "Buffer.vi"("Parameters"=w991, "Mode"=Buffer_state."Change Size", "Error IN"=w989) -> ("Error OUT"=w988:errorcluster)  [unwired: 4 in, 4 out]
        n319 = Merge Errors(w988) -> (w999:errorcluster)
      }
      frame "Exit" {
        # "Stop the VI"
        # "Exit - Send the Exit message to the UI Message Handler.  Call 'Flush Data to Log File.vi' so any pending data is not lost."
        n320 = Flush Queue(queue=w1007, error in (no error)=w1006) -> (error out=w1005:errorcluster)  [unwired: 2 out]
        n321 = call "Buffer.vi"("Mode"=Buffer_state."Exit", "Error IN"=w1005) -> ("Error OUT"=w1001:errorcluster)  [unwired: 5 in, 4 out]
        n322 = Unbundle By Name(w1003) -> ("Settings"=w1002:string)
        n323 = call "Save Settings to XML.vim"("error in (no error)"=w1001, "Settings File Name"=w1002, "Settings In"=w1003) -> ("error out"=w1000:errorcluster)  [unwired: 8 in]
        n324 = Merge Errors(w1000, w1006) -> (w1008:errorcluster)
      }
      frame "Flush" {
        n325 = call "Buffer.vi"("Mode"=Buffer_state."Flush", "Error IN"=w1012) -> ("Error OUT"=w1011:errorcluster)  [unwired: 5 in, 4 out]
      }
      frame "---Copy This Frame---" {
        # "Duplicate this frame when creating new messages.  Change this comment in the duplicated frame to describe this message."
        n326 = Merge Errors(w1016) -> (w1014:errorcluster)
      }
      frame Default {
        # "'Default' case only runs if there is a message that isn't defined in any of the other cases.  Output a programming error."
        n327 = xnode "Error Ring"("parameter 0"=w1017) -> ("error out"=w1018:errorcluster)
      }
    }
  }
  n328 = flat-sequence {
    tunnel: w20 -> [w1027]
    tunnel: [w1027] -> w18
    frame #0 {
      # "Add here the quitting sequence for your algorithm, if there are references to close for example"
    }
  }
  n329 = Merge Errors(w23, w32, w26, w25) -> (w24:errorcluster)
  n330 = Merge Errors(w24, w18) -> (w19:errorcluster)
  n331 = flat-sequence {
    tunnel: w33 -> [w1038]
    tunnel: w28 -> [w1035]
    tunnel: w27 -> [w1034]
    tunnel: w19 -> [w1031]
    tunnel: w21 -> [w1029]
    frame #0 {
      w1032 = TRUE ("force destroy? (F)")
      # "Quitting Sequence: Close all the references created in the template part"
      n332 = Unregister For Events(event registration refnum=w1038, error in=w1031) -> (error out=w1030:errorcluster)
      n333 = call "Destroy User Event - Stop.vi"("error in (no error)"=w1030, "User Event - Stop"=w1029) -> ("error out"=w1036:errorcluster)  [unwired: 9 in]
      n334 = Cluster To Array(cluster=w1034) -> (array=w1037:refnum<queue>[])
      n335 = for {
        shift-right: [w1042] -> w1028
        shift-left: w1036 -> [w1041]
        tunnel: w1032 -> [w1040]
        tunnel: w1037 -> [w1039] mode=indexing
        n336 = Release Queue(queue=w1039, force destroy? (F)=w1040, error in (no error)=w1041) -> (error out=w1042:errorcluster)  [unwired: 2 out]
      }
      n337 = Release Queue(queue=w1035, force destroy? (F)=w1032, error in (no error)=w1028) -> (error out=w1033:errorcluster)  [unwired: 2 out]
      n338 = disable-structure shown="RUN_TIME_ENGINE==True" {
        disable-tunnel: w1033 -> [_ _]
        frame condition #0 (active) {
        }
        frame condition #1 {
          # "Call Quit LabVIEW if running as a built application."
          n339 = Quit LabVIEW() -> ()  [unwired: 1 in]
        }
      }
    }
  }
